vi "Autonomous Independent.vi"() -> ()   [LabVIEW 2020]
doc: "This VI is called when autonomous begins, and will automatically be terminated when autonomous ends. You can carry out timed or sensor driven robot movement independently without needing to return to the caller."
uses:
  <vilib>/Rock Robotics/WPI/Solenoid/WPI_SolenoidValue.ctl
  <vilib>/Rock Robotics/WPI/Utilities/WPI_GetSetVariantRefNum.vi
  <vilib>/Rock Robotics/Network Tables/NT Write Numeric Array.vi
  <vilib>/Rock Robotics/WPI/Solenoid/WPI_SolenoidSetEnum.vi
  Robot Global Data.vi
  <vilib>/Rock Robotics/WPI/RobotDrive/WPI_RobotDriveArcadeDrive_Standard(NoSaturation).vi
  <vilib>/Rock Robotics/Network Tables/NT Read String.vi
panel:
  out "Current Movement, for debugging":T1 {"Y Joystick Value" scale=1.0..-1.0; "X Joystick Value" scale=-1.0..1.0}
  in  "Array of robot movements":T2(array[cluster])=[{"X Joystick Value"=0.39393939393939403, "Y Joystick Value"=0.0, "Delay (sec)"=1.0, "Movement Name"="turn"}, {"X Joystick Value"=-0.3737373737373737, "Y Joystick Value"=0.0, "Delay (sec)"=1.0, "Movement Name"="turn back"}] {"Y Joystick Value" scale=1.0..-1.0; "X Joystick Value" scale=-1.0..1.0}
  # "Be sure to right-click and choose Data Operations>>Make Current Value default if you want to save the array values with the VI"
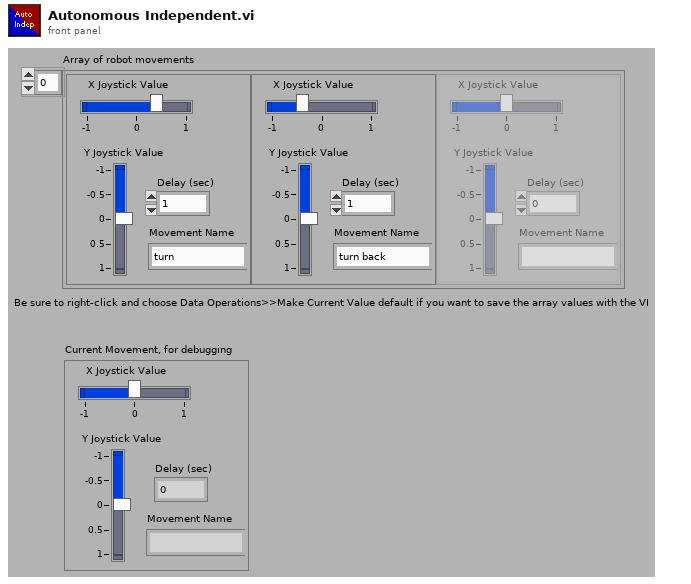
[diagram p1: front panel]
types:
  T1 = cluster{"X Joystick Value":dbl, "Y Joystick Value":dbl, "Delay (sec)":dbl, "Movement Name":string}
  T2 = cluster{"X Joystick Value":dbl, "Y Joystick Value":dbl, "Delay (sec)":dbl, "Movement Name":string}[]
  T3 = typedef "WPI_JoystickDevRef.ctl" = cluster{"Device":T4}
  T4 = typedef "WPI_JoystickDeviceEnum.ctl" = enum16{"USB 0", "USB 1", "USB 2", "USB 3", "USB 4", "USB 5"}
  T5 = typedef "WPI_SolenoidValue.ctl" = enum16{"Off", "On", "Forward", "Reverse"}
  T6 = typedef "WPI_MotorControlDeviceRef.ctl" = cluster{"DeviceStatus":errorcluster, "Type":T7, "PWM":cluster{"PWM Channel":T8, "DeadBand":T9}, "CAN":cluster{"Device Number":u8, "SetOutput VI Ref":variant, "GetOutput VI Ref":variant, "Enable VI Ref":variant, "Disable VI Ref":variant, "Data":variant}, "Invert":bool, "DIO PWM":cluster{"PWM \"Enable\" Channel":T8, "DIOChannel":T10, "PWM Rate":dbl}}
  T7 = typedef "WPI_MotorControlType.ctl" = enum16{"PWM", "CAN", "DIO PWM"}
  T8 = typedef "FPGA_DIOPWMChannel.ctl" = enum8{"PWM 0", "PWM 1", "PWM 2", "PWM 3", "PWM 4", "PWM 5", "PWM 6", "PWM 7", "PWM 8", "PWM 9", "PWM MXP 0", "PWM MXP 1", "PWM MXP 2", "PWM MXP 3", "PWM MXP 4", "PWM MXP 5", "PWM MXP 6", "PWM MXP 7", "PWM MXP 8", "PWM MXP 9", "Invalid"}
  T9 = typedef "WPI_PWMDeadband.ctl" = cluster{"Name":string, "maxPositivePwm":i32, "minPositivePwm":i32, "centerPwm":i32, "maxNegativePwm":i32, "minNegativePwm":i32, "angularRange":u16}
  T10 = typedef "FPGA_DIOChannel.ctl" = enum8{"DIO 0", "DIO 1", "DIO 2", "DIO 3", "DIO 4", "DIO 5", "DIO 6", "DIO 7", "DIO 8", "DIO 9", "DIO MXP 0", "DIO MXP 1", "DIO MXP 2", "DIO MXP 3", "DIO MXP 4", "DIO MXP 5", "DIO MXP 6", "DIO MXP 7", "DIO MXP 8", "DIO MXP 9", "DIO MXP 10", "DIO MXP 11", "DIO MXP 12", "DIO MXP 13", "DIO MXP 14", "DIO MXP 15", "SPI Port CS1", "SPI Port CS2", "SPI Port CS3", "SPI Port MISO", "SPI Port MOSI", "Invalid"}
  T11 = typedef "WPI_SolenoidDevRef.ctl" = cluster{"DevStatus":errorcluster, "Pneumatics Control Module":u8, "Forward Solenoid Channel":T12, "Reverse Solenoid Channel":T12}
  T12 = typedef "WPI_SolenoidChannel.ctl" = enum8{"Solenoid 0", "Solenoid 1", "Solenoid 2", "Solenoid 3", "Solenoid 4", "Solenoid 5", "Solenoid 6", "Solenoid 7", "Solenoid 8", "Solenoid 9", "Solenoid 10", "Solenoid 11", "Solenoid 12", "Solenoid 13", "Solenoid 14", "Solenoid 15", "Invalid"}
  T13 = typedef "WPI_RobotDriveDevRef.ctl" = cluster{"DevStatus":errorcluster, "Motors[]":T6[], "Square Inputs":bool, "Max Output":dbl}
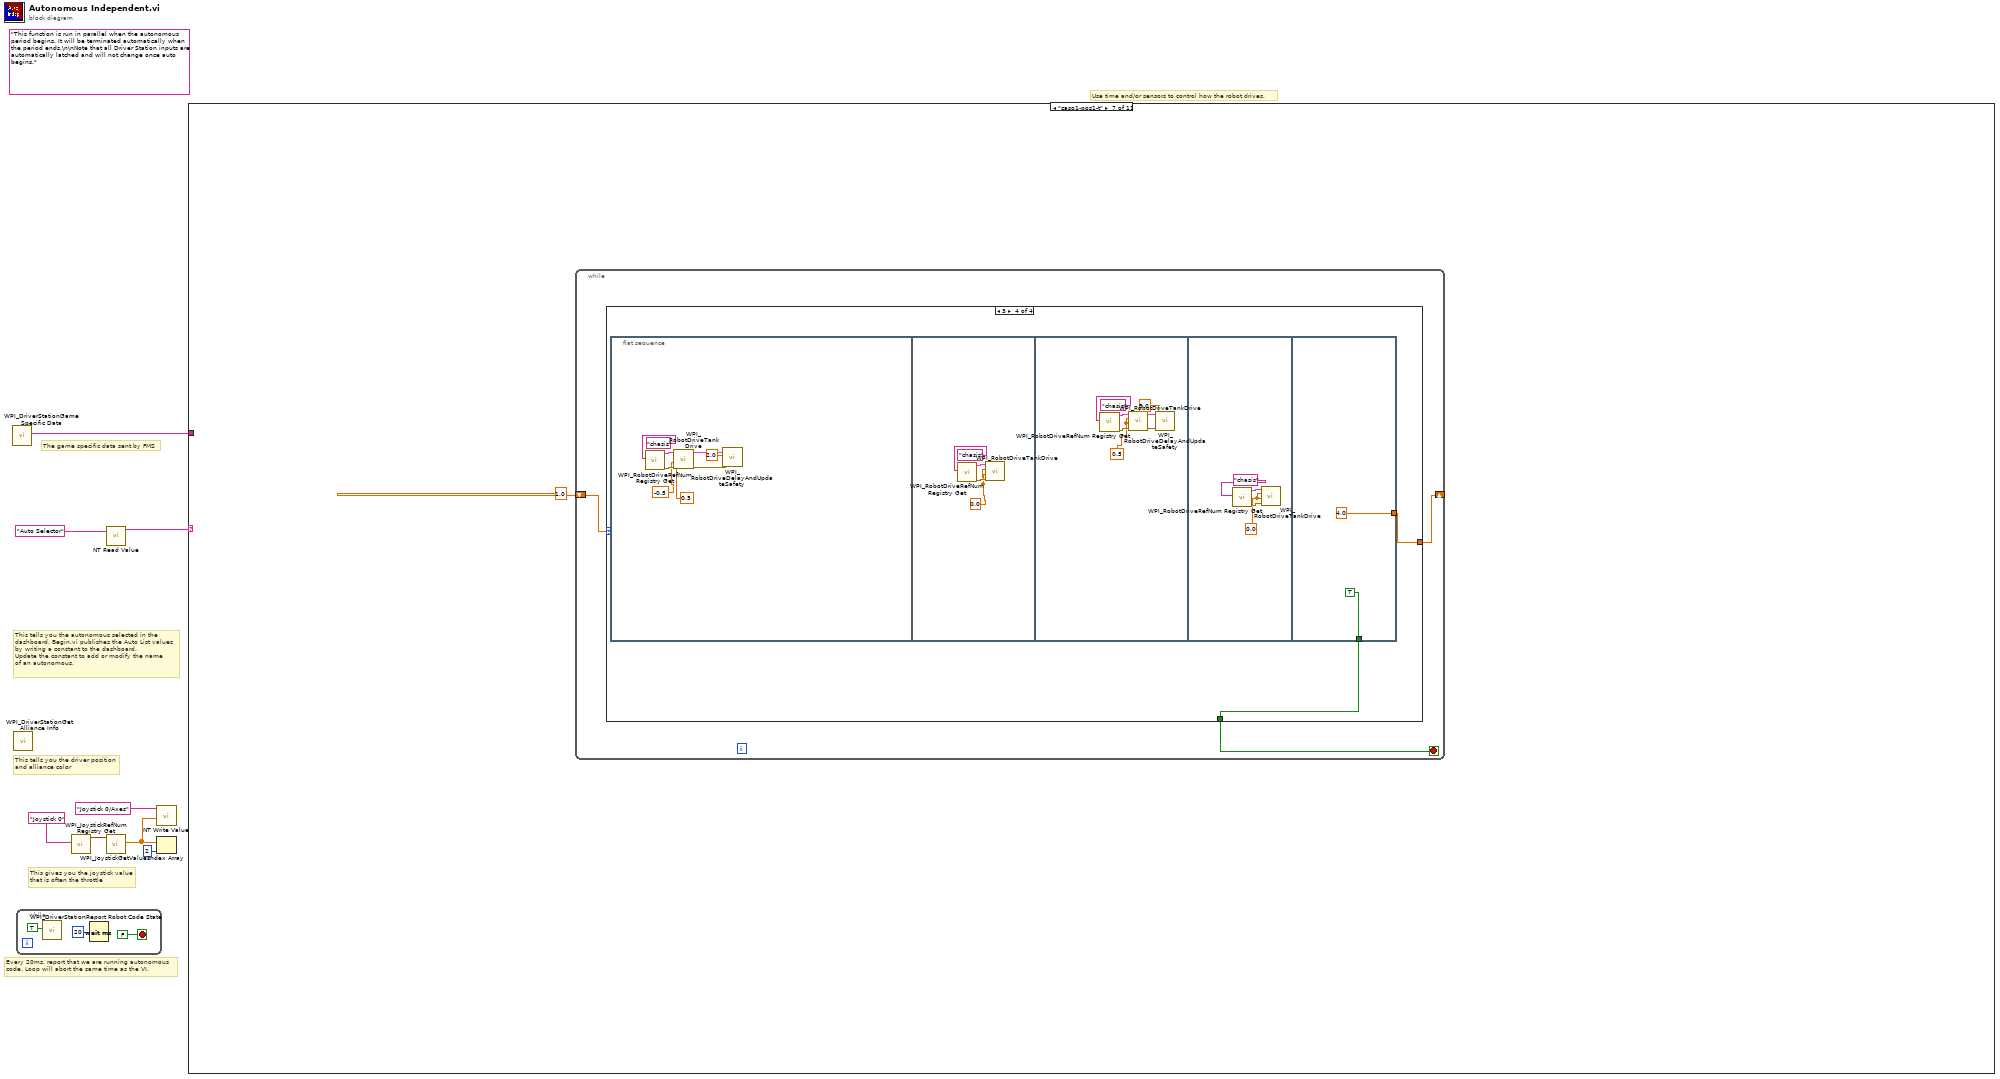
[diagram p0: block diagram]
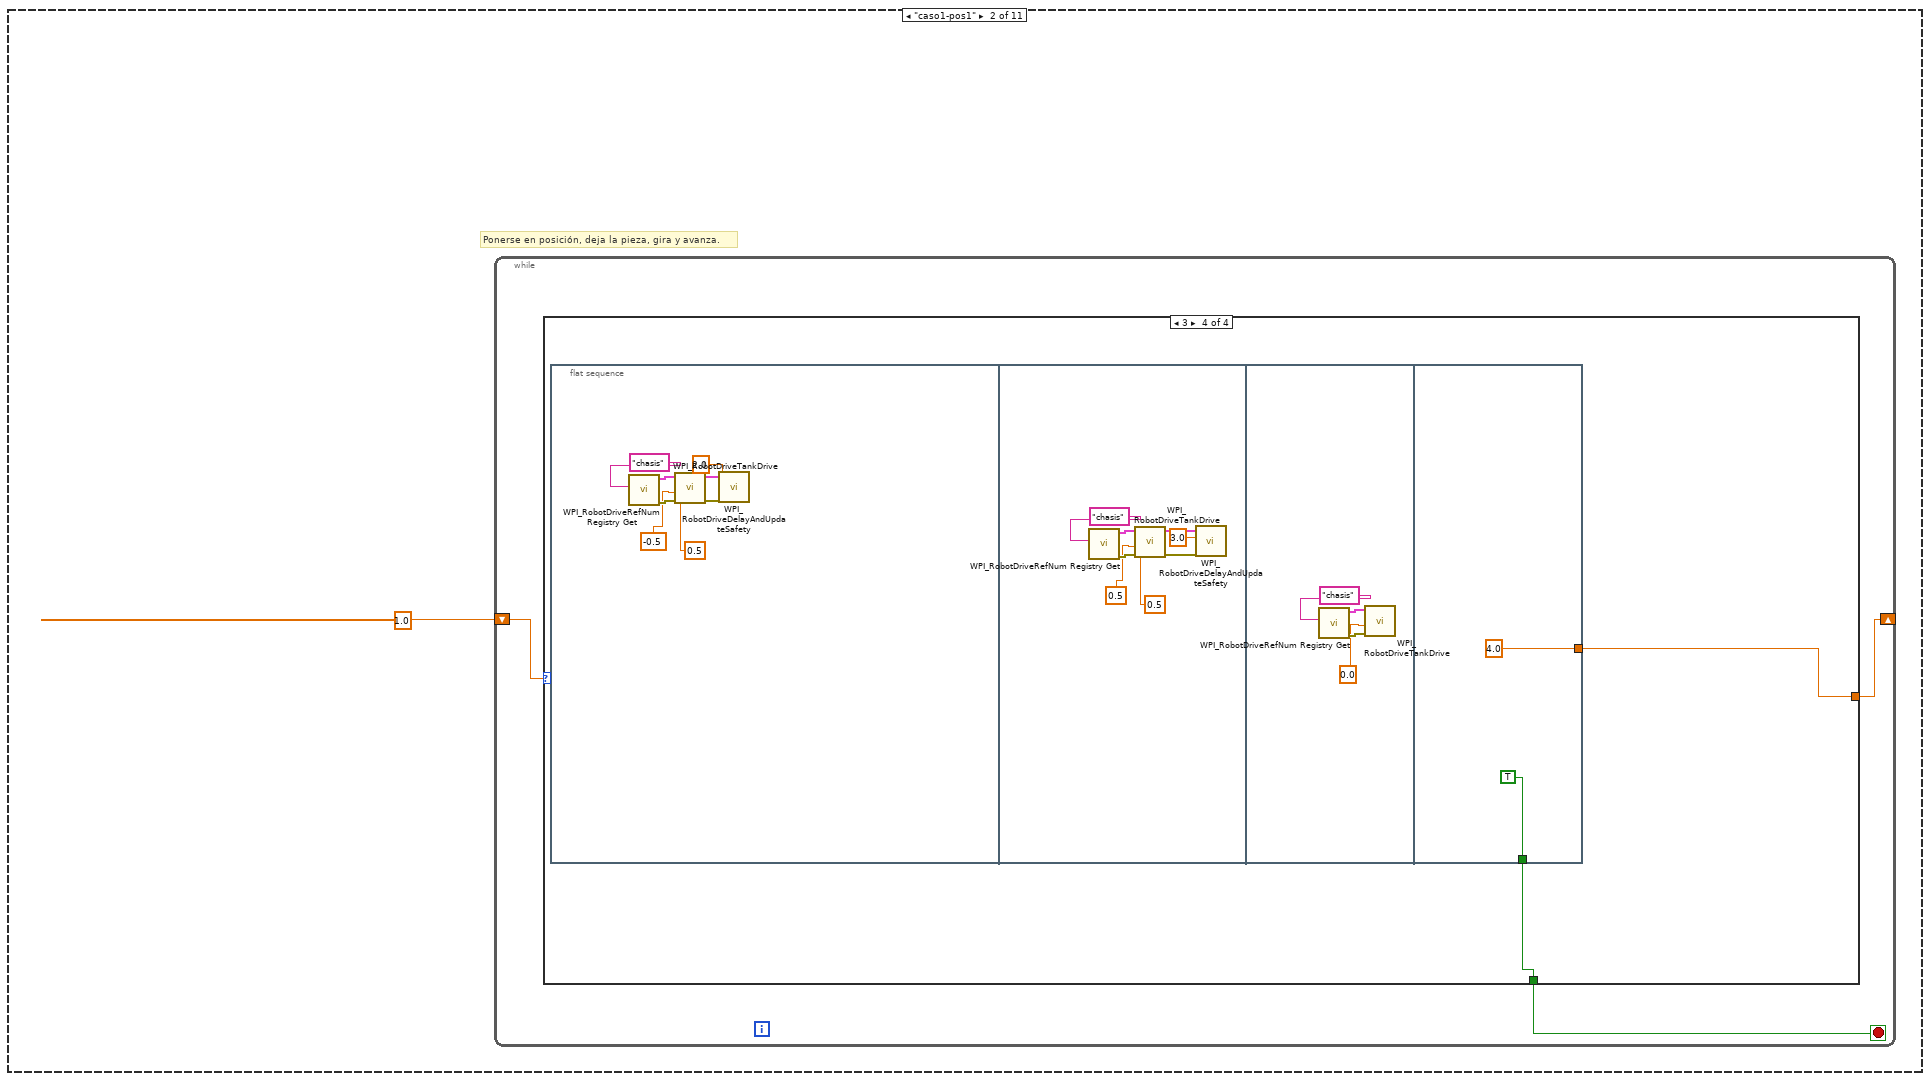
[diagram p3: hidden frame]
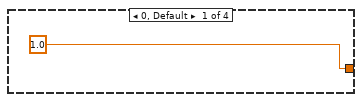
[diagram p4: hidden frame]
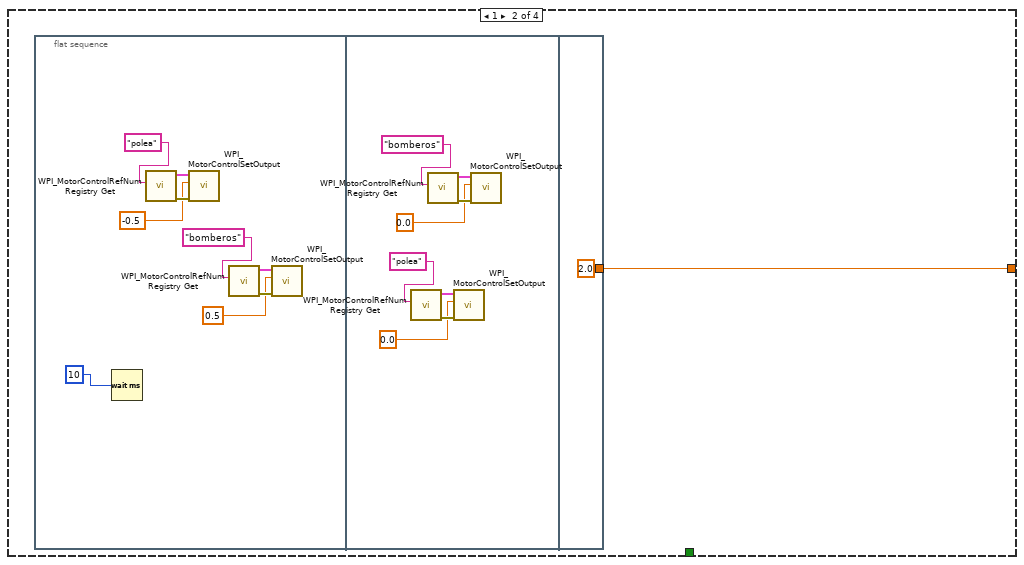
[diagram p5: hidden frame]
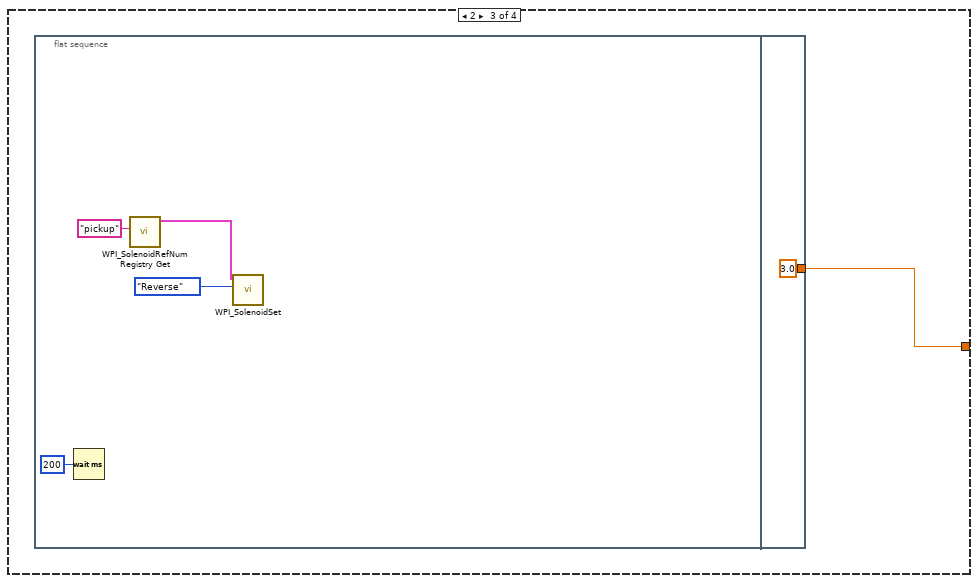
[diagram p6: hidden frame]
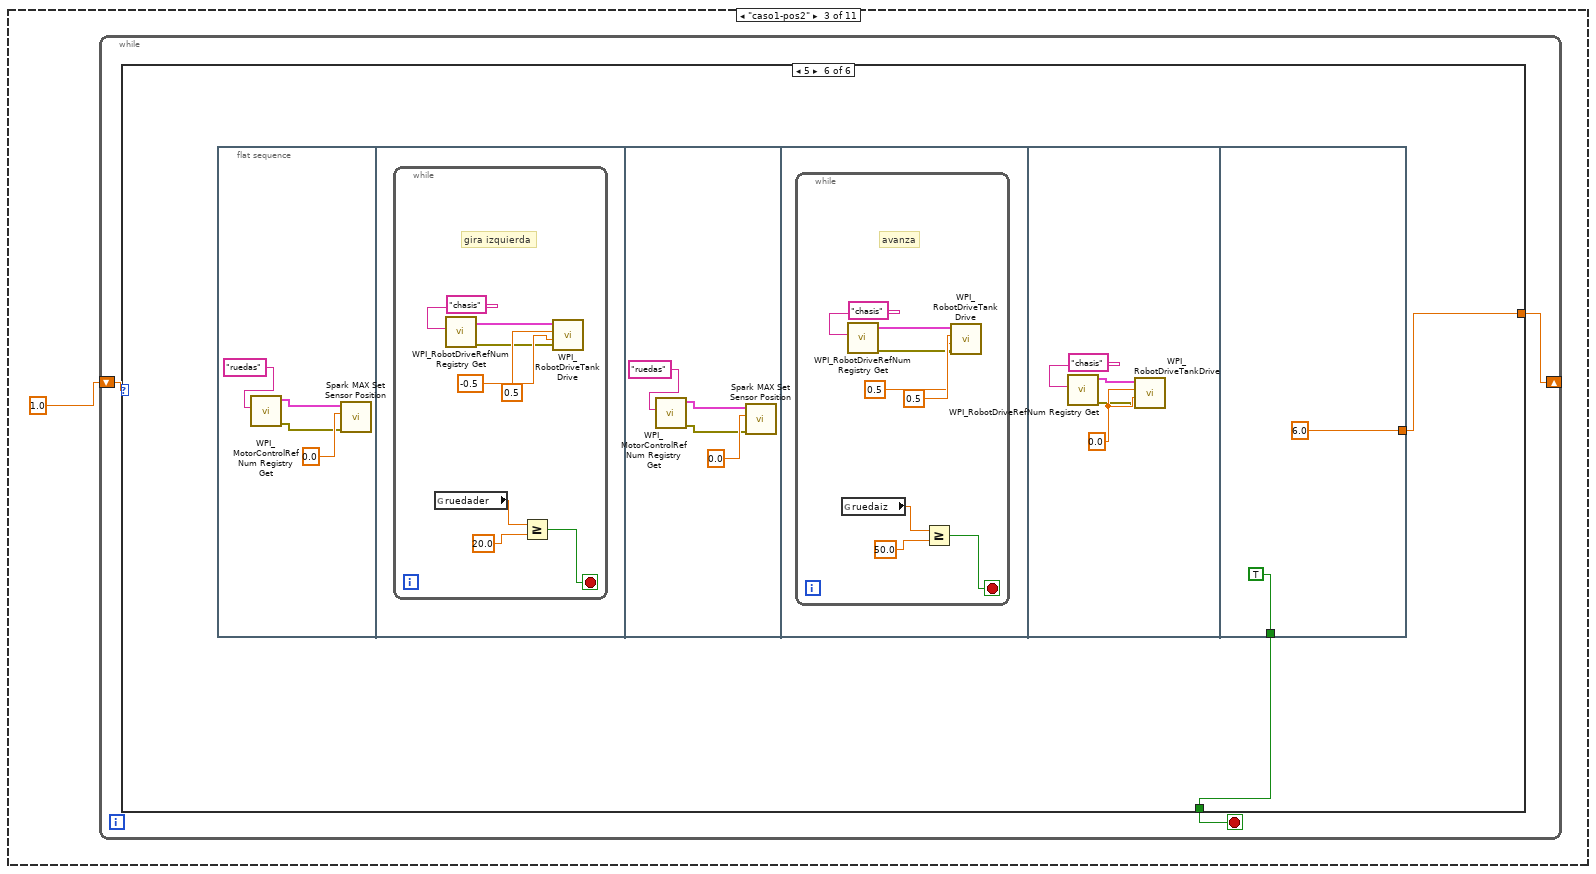
[diagram p7: hidden frame]
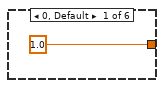
[diagram p8: hidden frame]
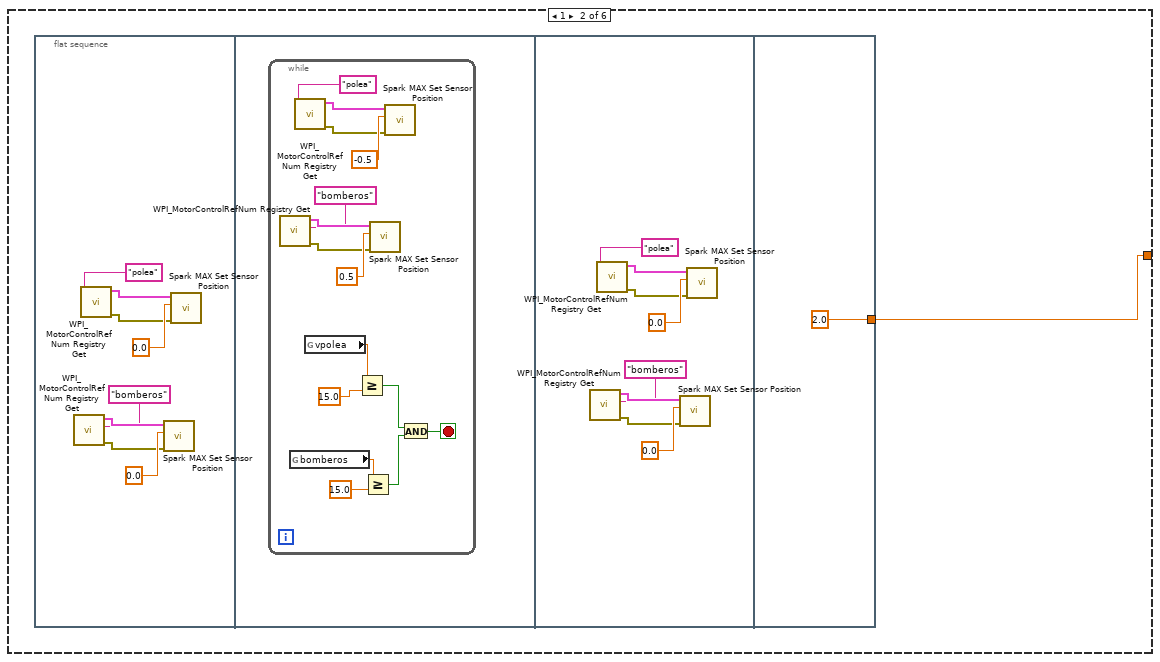
[diagram p9: hidden frame]
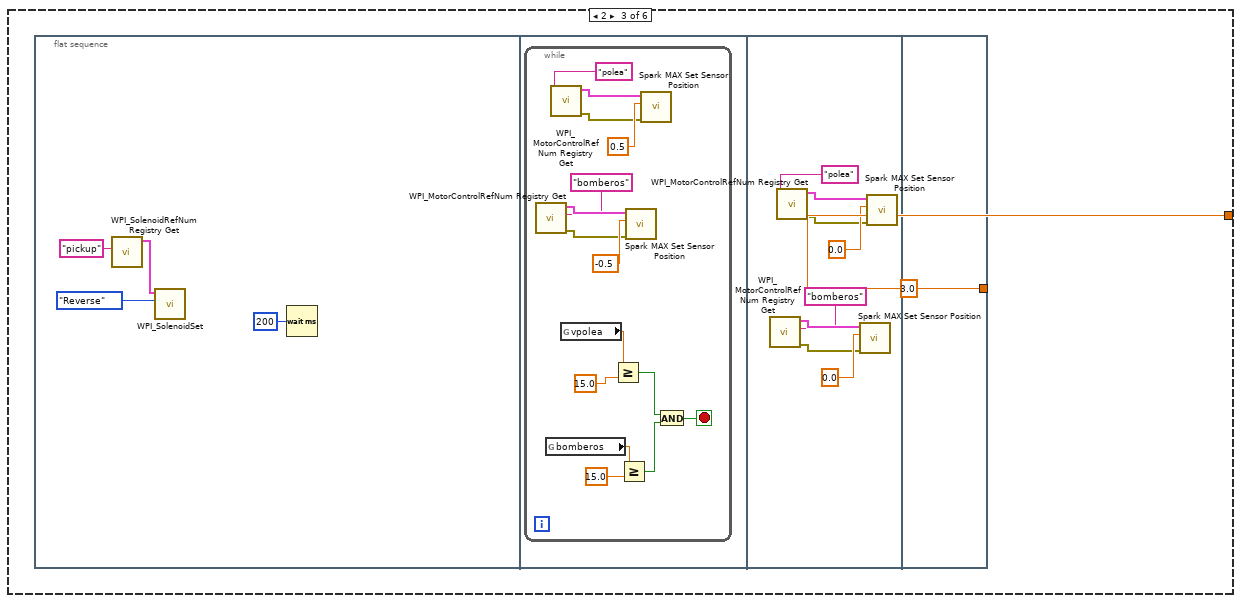
[diagram p10: hidden frame]
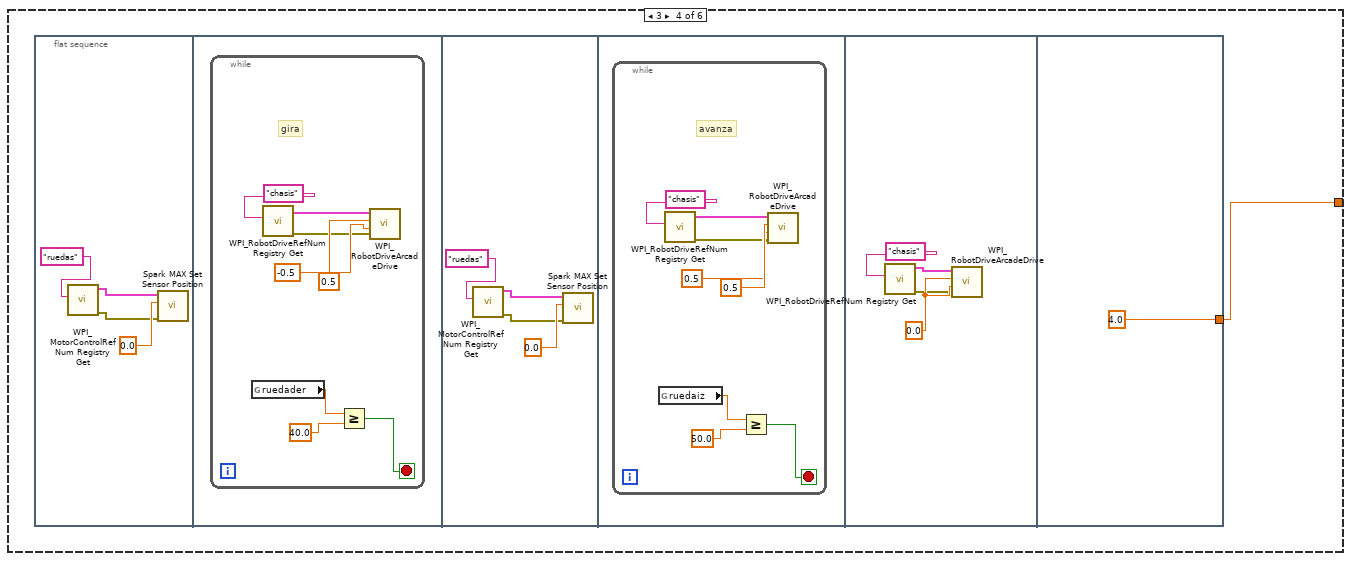
[diagram p11: hidden frame]
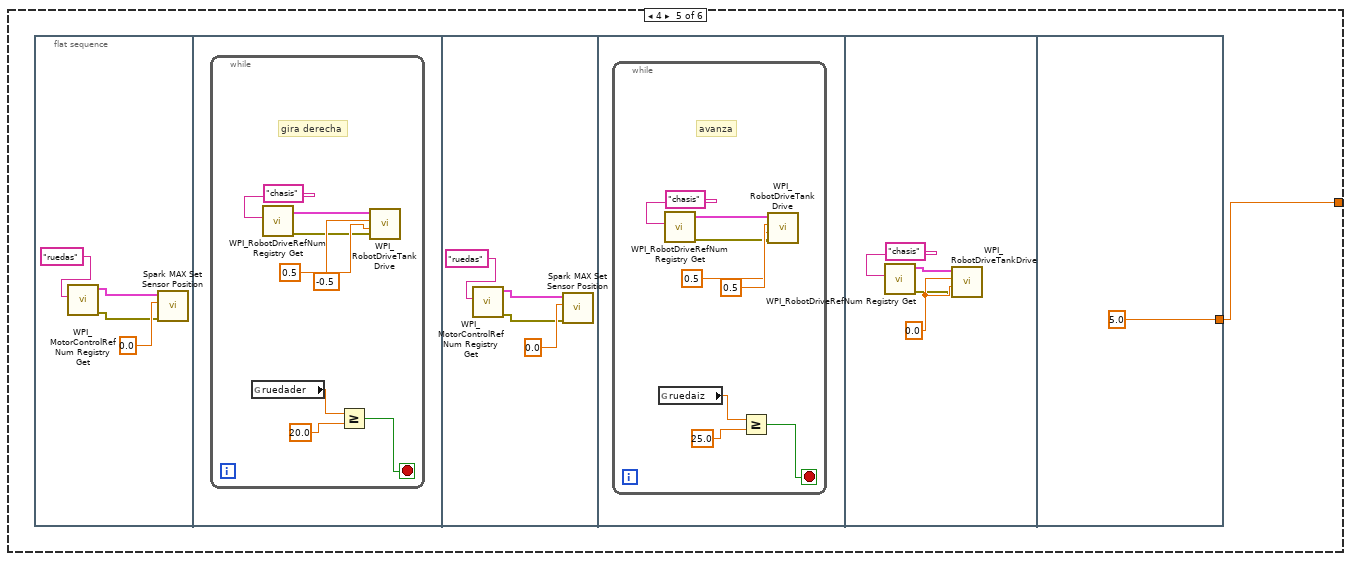
[diagram p12: hidden frame]
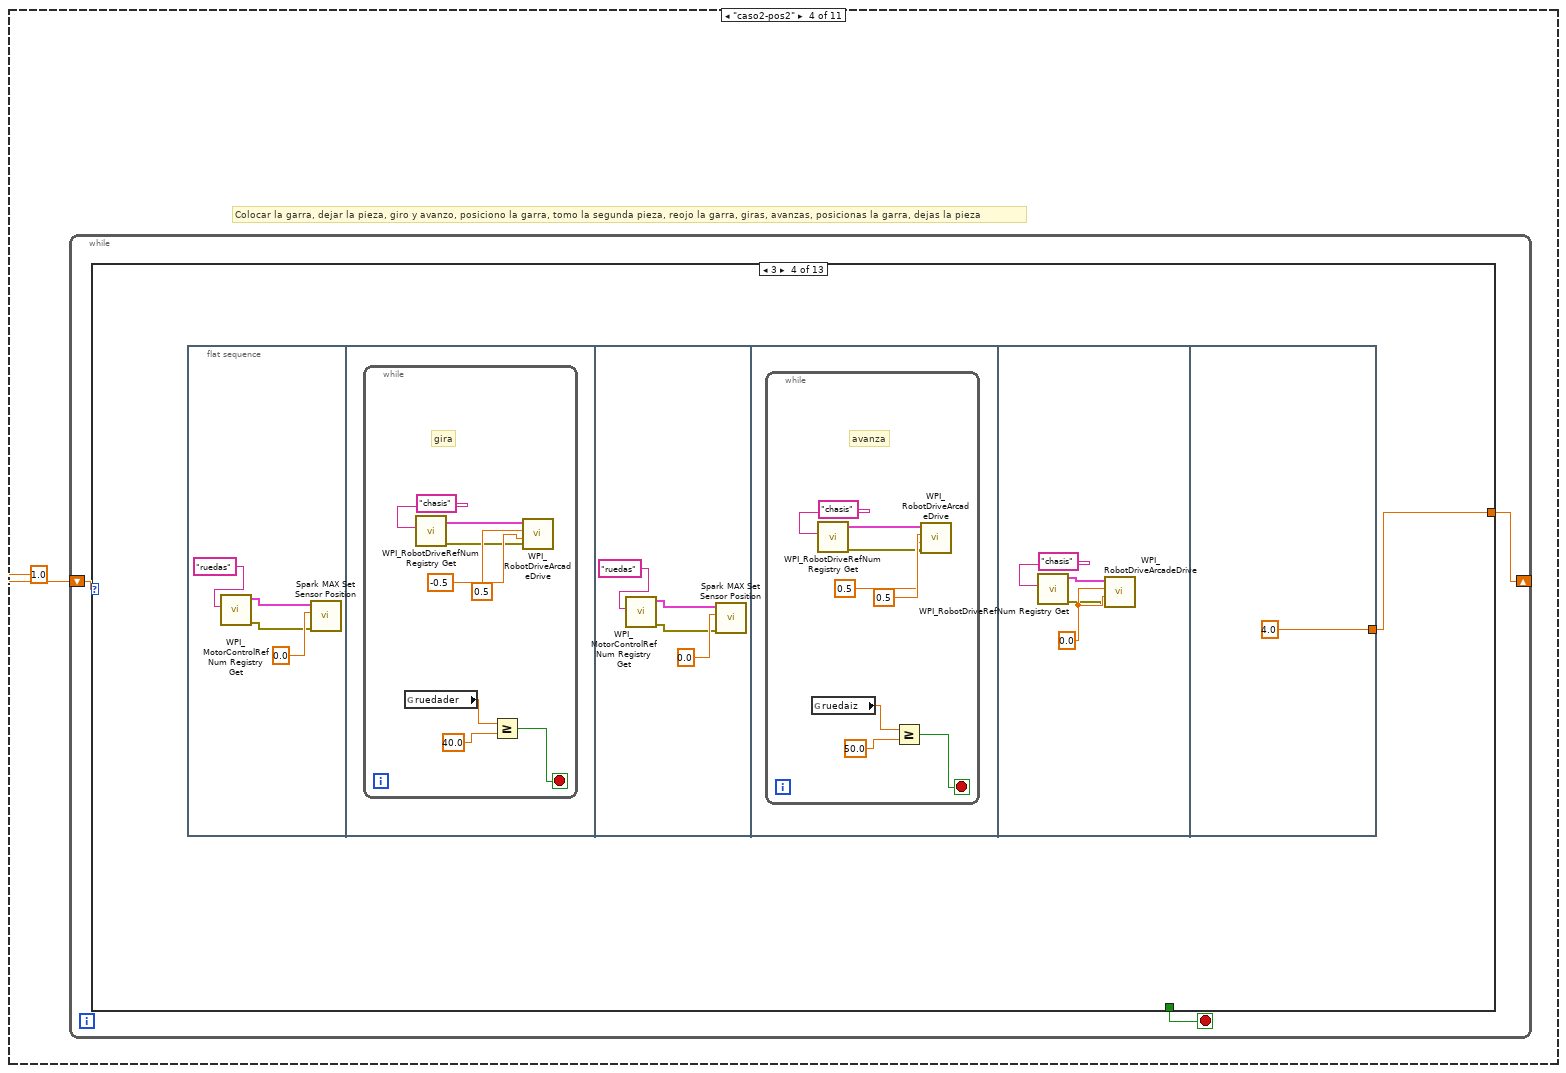
[diagram p13: hidden frame]
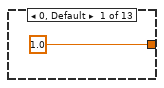
[diagram p14: hidden frame]
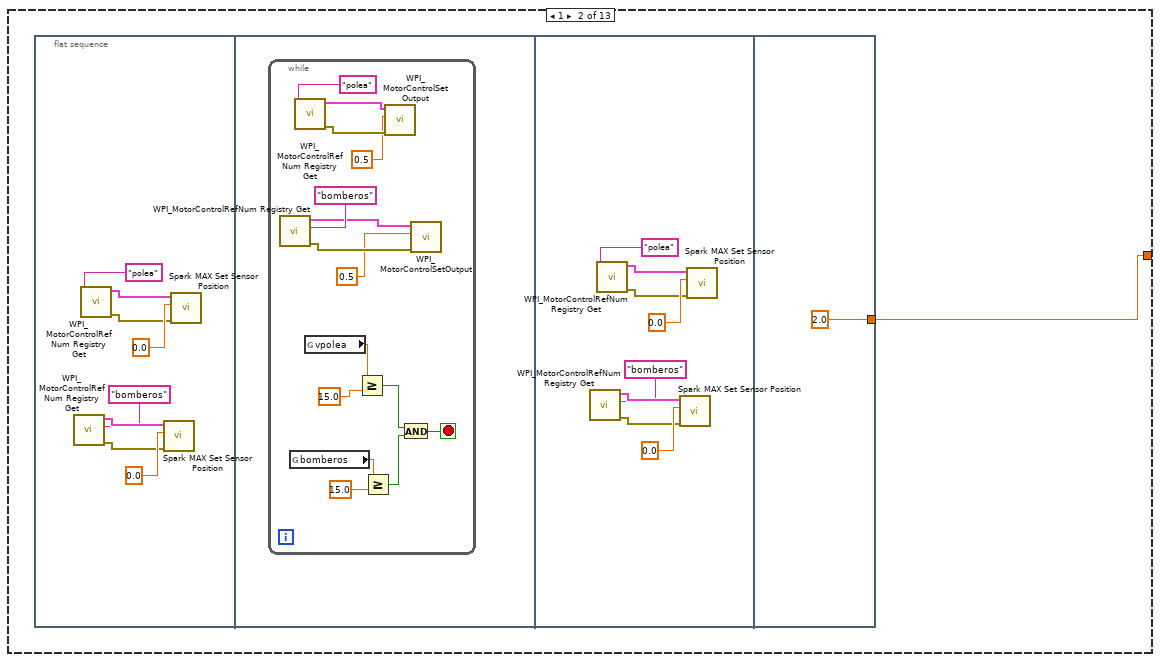
[diagram p15: hidden frame]
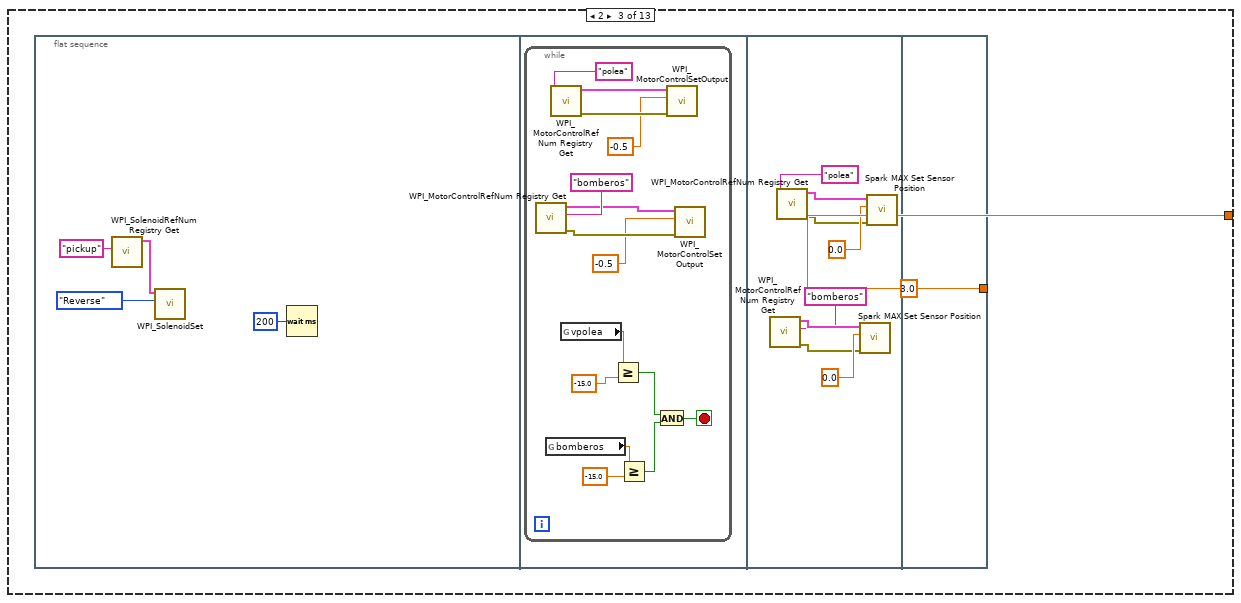
[diagram p16: hidden frame]
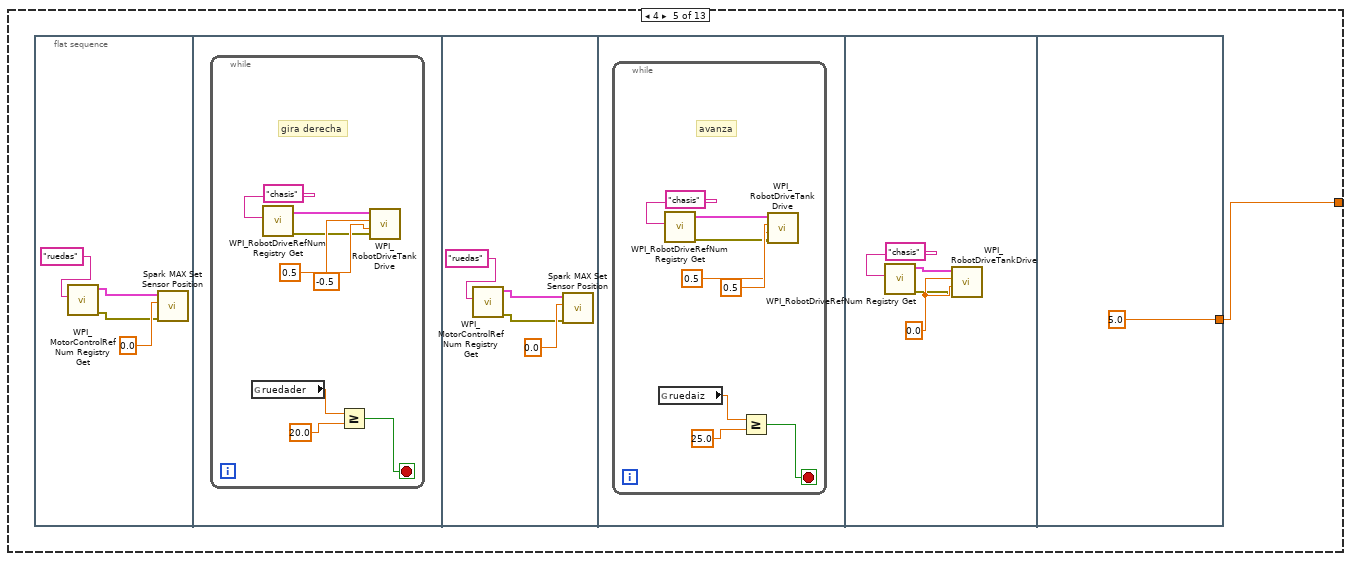
[diagram p17: hidden frame]
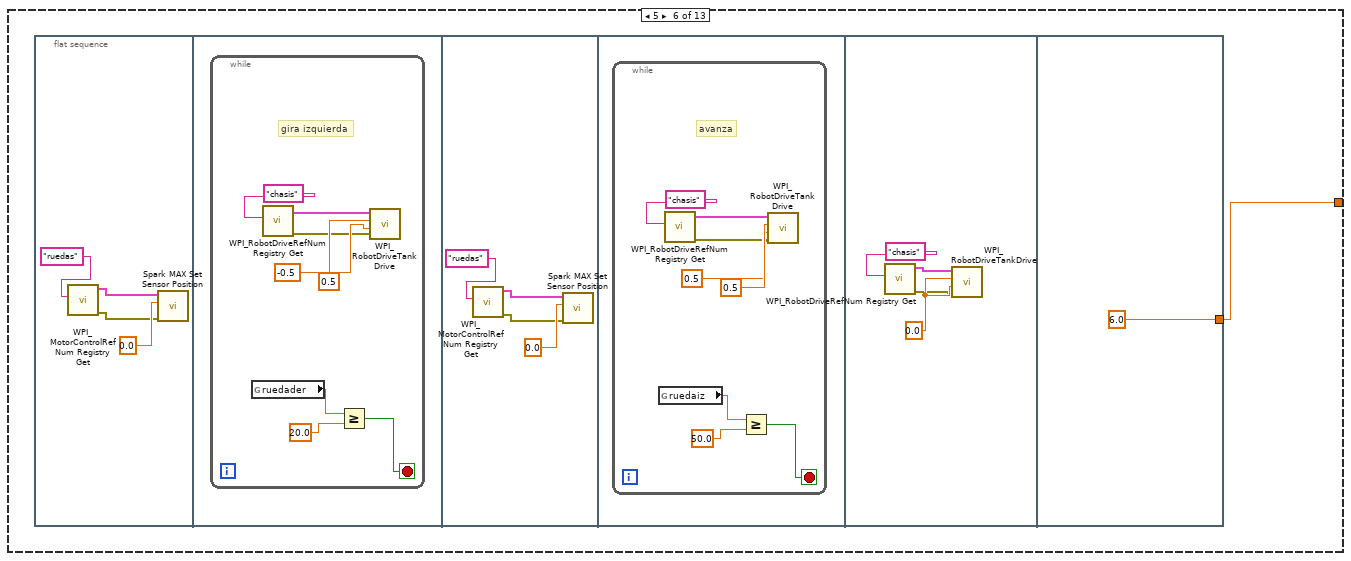
[diagram p18: hidden frame]
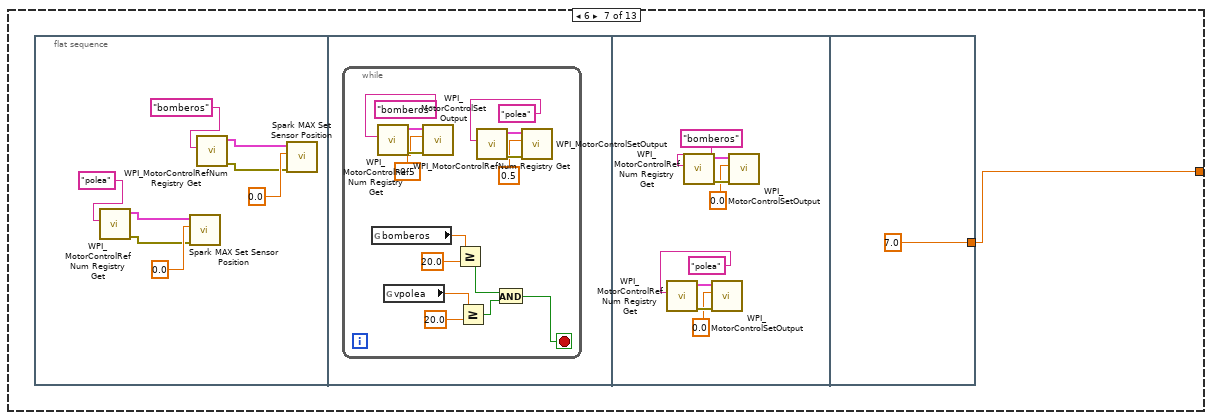
[diagram p19: hidden frame]
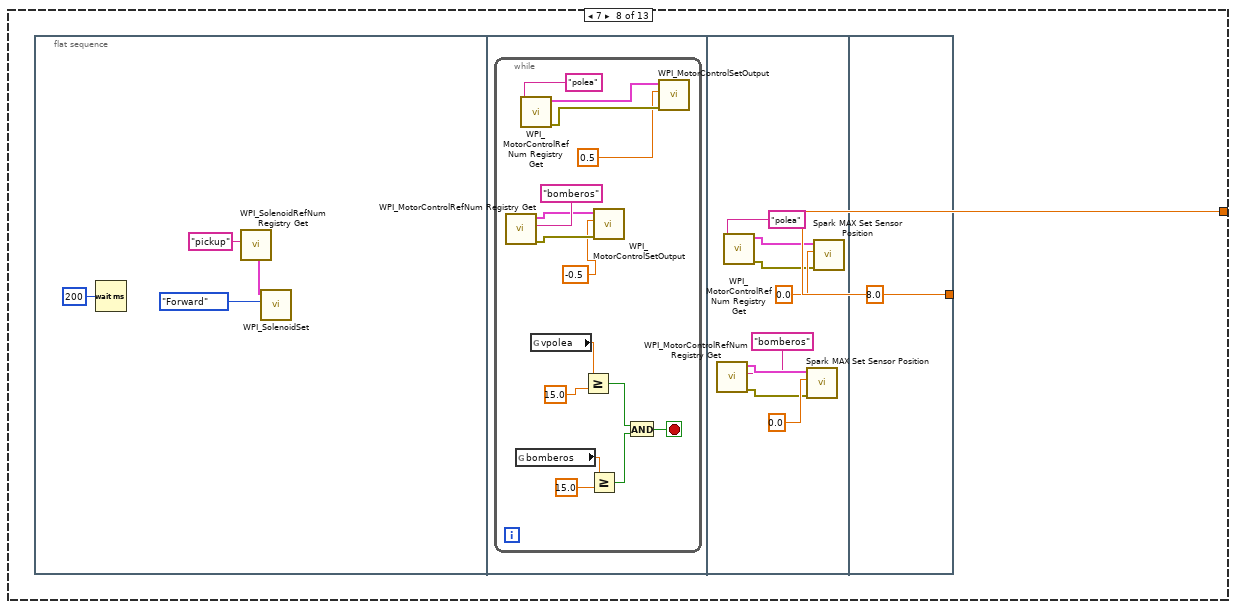
[diagram p20: hidden frame]
diagram:
  (unwired) "This function is run in parallel when the autonomous period begins. It will be terminated automatically when the period ends.\n\nNote that all Driver Station inputs are automatically latched and will not change once auto begins."
  # "The game specific data sent by FMS"
  # "This tells you the autonomous selected in the \ndashboard. Begin.vi publishes the Auto List values\nby writing a constant to the dashboard.\nUpdate the constant to add or modify the name\nof an autonomous."
  # "Every 20ms, report that we are running autonomous\ncode. Loop will abort the same time as the VI."
  # "This gives you the joystick value\nthat is often the throttle"
  # "Use time and/or sensors to control how the robot drives."
  # "This tells you the driver position\nand alliance color"
  n1 = call <vilib>:"WPI_DriverStationGame Specific Data.vi"() -> ("Game Specific Data"=w1:string)  [unwired: 11 in]
  n2 = call <vilib>:"WPI_DriverStationGet Alliance Info.vi"() -> ()  [unwired: 12 out]
  n3 = while {
    stop <- FALSE stop-if-true
    n4 = call <vilib>:"WPI_DriverStationReport Robot Code State.vi"("Autonomous"=TRUE) -> ()  [unwired: 10 in, 1 out]
    n5 = Wait (ms)(milliseconds to wait=u32 20) -> ()  [unwired: 1 out]
  }
  n6 = call <vilib>:"WPI_JoystickRefNum Registry Get.vi"("refnum name"="Joystick 0") -> ("JoystickDevRef"=w7:T3)  [unwired: 1 in, 9 out]
  n7 = call <vilib>:"WPI_JoystickGetValues.vi"("JoystickDevRef"=w7) -> ("Axes"=w3:dbl[])  [unwired: 6 in, 4 out]
  n8 = call-poly <vilib>:"NT Read Value.vi"("Name"="Auto Selector") -> ("String"=w4:string)  [unwired: 9 in, 1 out]
  n9 = call-poly <vilib>:"NT Write Value.vi"("Numeric Array"=w3, "Name"="Joystick 0/Axes") -> ()  [unwired: 9 in, 1 out]
  n10 = Index Array(array=w3, index=2) -> ()  [unwired: 1 out]
  n11 = case shown="\"caso1-pos1-t\"" w4 {
    tunnel: w1 -> [_ _ _ _ _ _ _ _ _ _ _]
    frame Default {
      # "You can put your main auto here, or you can right-click on the case and make any\nother frame be the default case."
      # "This is the frame that will execute if no selection is made, or if it is not recognized"
    }
    frame "caso1-pos1" {
      # "Ponerse en posición, deja la pieza, gira y avanza."
      n12 = while {
        shift-right: [w15] -> _
        shift-left: 1.0 -> [w13]
        stop <- w14 stop-if-true
        n13 = case shown="3" w13 {
          tunnel: [1.0 w17 w36 w43] -> w15
          tunnel: [_ _ _ w42] -> w14
          frame 0, Default {
          }
          frame 1 {
            n14 = flat-sequence {
              tunnel: [2.0] -> w17
              frame #0 {
                n15 = Wait (ms)(milliseconds to wait=u32 10 ("millisecond timer value")) -> ()  [unwired: 1 out]
                n16 = call <vilib>:"WPI_MotorControlRefNum Registry Get.vi"("refnum name"="polea") -> ("error out"=w26:errorcluster, "MotorControlDevRef"=w25:T6)  [unwired: 9 in]
                n17 = call <vilib>:"WPI_MotorControlSetOutput.vi"("error in (no error)"=w26, "Output"=-0.5, "MotorControlDevRef"=w25) -> ()  [unwired: 6 in, 3 out]
                n18 = call <vilib>:"WPI_MotorControlRefNum Registry Get.vi"("refnum name"="bomberos") -> ("error out"=w22:errorcluster, "MotorControlDevRef"=w21:T6)  [unwired: 9 in]
                n19 = call <vilib>:"WPI_MotorControlSetOutput.vi"("error in (no error)"=w22, "Output"=0.5, "MotorControlDevRef"=w21) -> ()  [unwired: 6 in, 3 out]
              }
              frame #1 {
                n20 = call <vilib>:"WPI_MotorControlRefNum Registry Get.vi"("refnum name"="polea") -> ("error out"=w33:errorcluster, "MotorControlDevRef"=w34:T6)  [unwired: 9 in]
                n21 = call <vilib>:"WPI_MotorControlRefNum Registry Get.vi"("refnum name"="bomberos") -> ("error out"=w29:errorcluster, "MotorControlDevRef"=w30:T6)  [unwired: 9 in]
                n22 = call <vilib>:"WPI_MotorControlSetOutput.vi"("error in (no error)"=w33, "Output"=0.0, "MotorControlDevRef"=w34) -> ()  [unwired: 6 in, 3 out]
                n23 = call <vilib>:"WPI_MotorControlSetOutput.vi"("error in (no error)"=w29, "Output"=0.0, "MotorControlDevRef"=w30) -> ()  [unwired: 6 in, 3 out]
              }
              frame #2 {
              }
            }
          }
          frame 2 {
            n24 = flat-sequence {
              tunnel: [3.0] -> w36
              frame #0 {
                n25 = Wait (ms)(milliseconds to wait=u32 200) -> ()  [unwired: 1 out]
                n26 = call <vilib>:"WPI_SolenoidRefNum Registry Get.vi"("refnum name"="pickup") -> ("SolenoidDevRef"=w40:T11)  [unwired: 9 in, 1 out]
                n27 = call-poly <vilib>:"WPI_SolenoidSet.vi"("Value"=WPI_SolenoidValue."Reverse", "SolenoidDevRef"=w40) -> ()  [unwired: 8 in, 2 out]
              }
              frame #1 {
              }
            }
          }
          frame 3 {
            n28 = flat-sequence {
              tunnel: [4.0] -> w43
              tunnel: [TRUE] -> w42
              frame #0 {
                n29 = call <vilib>:"WPI_RobotDriveRefNum Registry Get.vi"("refnum name"="chasis") -> ("error out"=w51:errorcluster, "RobotDriveDevRef"=w50:T13)  [unwired: 9 in]
                n30 = call <vilib>:"WPI_RobotDriveTankDrive.vi"("error in (no error)"=w51, "Right axis value"=-0.5 ("Motor Output"), "Left axis value"=0.5 ("Motor Output"), "RobotDriveDevRef"=w50) -> ("error out"=w46:errorcluster, "RobotDriveDevRef"=w45:T13)  [unwired: 5 in, 1 out]
                n31 = call <vilib>:"WPI_RobotDriveDelayAndUpdateSafety.vi"("error in (no error)"=w46, "Delay (s)"=2.0, "RobotDriveDevRef"=w45) -> ()  [unwired: 7 in, 2 out]
              }
              frame #1 {
                n32 = call <vilib>:"WPI_RobotDriveRefNum Registry Get.vi"("refnum name"="chasis") -> ("error out"=w59:errorcluster, "RobotDriveDevRef"=w58:T13)  [unwired: 9 in]
                n33 = call <vilib>:"WPI_RobotDriveTankDrive.vi"("error in (no error)"=w59, "Right axis value"=0.5 ("Motor Output"), "Left axis value"=0.5 ("Motor Output"), "RobotDriveDevRef"=w58) -> ("error out"=w53:errorcluster, "RobotDriveDevRef"=w54:T13)  [unwired: 5 in, 1 out]
                n34 = call <vilib>:"WPI_RobotDriveDelayAndUpdateSafety.vi"("error in (no error)"=w53, "Delay (s)"=3.0, "RobotDriveDevRef"=w54) -> ()  [unwired: 7 in, 2 out]
              }
              frame #2 {
                n35 = call <vilib>:"WPI_RobotDriveRefNum Registry Get.vi"("refnum name"="chasis") -> ("error out"=w63:errorcluster, "RobotDriveDevRef"=w62:T13)  [unwired: 9 in]
                n36 = call <vilib>:"WPI_RobotDriveTankDrive.vi"("error in (no error)"=w63, "Right axis value"=0.0 ("Motor Output"), "RobotDriveDevRef"=w62) -> ()  [unwired: 6 in, 3 out]
              }
              frame #3 {
              }
            }
          }
        }
      }
    }
    frame "caso1-pos2" {
      n37 = while {
        shift-right: [w68] -> _
        shift-left: 1.0 -> [w69]
        stop <- w67 stop-if-true
        n38 = case shown="5" w69 {
          tunnel: [1.0 w71 w104 w133 w163 w194] -> w68
          tunnel: [_ _ _ _ _ w193] -> w67
          frame 0, Default {
          }
          frame 1 {
            n39 = flat-sequence {
              tunnel: [2.0] -> w71
              frame #0 {
                n40 = call <vilib>:"WPI_MotorControlRefNum Registry Get.vi"("refnum name"="bomberos") -> ("error out"=w74:errorcluster, "MotorControlDevRef"=w75:T6)  [unwired: 9 in]
                n41 = call <vilib>:"WPI_MotorControlRefNum Registry Get.vi"("refnum name"="polea") -> ("error out"=w77:errorcluster, "MotorControlDevRef"=w78:T6)  [unwired: 9 in]
                n42 = call <vilib>:"Spark MAX Set Sensor Position.vi"("error in"=w74, "Position"=0.0, "MotorControlDeviceRef"=w75) -> ()  [unwired: 7 in, 2 out]
                n43 = call <vilib>:"Spark MAX Set Sensor Position.vi"("error in"=w77, "Position"=0.0, "MotorControlDeviceRef"=w78) -> ()  [unwired: 7 in, 2 out]
              }
              frame #1 {
                n44 = while {
                  stop <- w92 stop-if-true
                  n45 = call <vilib>:"WPI_MotorControlRefNum Registry Get.vi"("refnum name"="bomberos") -> ("error out"=w84:errorcluster, "MotorControlDevRef"=w85:T6)  [unwired: 9 in]
                  n46 = global read "Robot Global Data.vi" "bomberos"() -> (w91:dbl)
                  n47 = call <vilib>:"WPI_MotorControlRefNum Registry Get.vi"("refnum name"="polea") -> ("error out"=w87:errorcluster, "MotorControlDevRef"=w88:T6)  [unwired: 9 in]
                  n48 = global read "Robot Global Data.vi" "vpolea"() -> (w94:dbl)
                  n49 = Greater Or Equal?(x=w94, y=15.0) -> (x >= y?=w81:bool)
                  n50 = Greater Or Equal?(x=w91, y=15.0) -> (x >= y?=w80:bool)
                  n51 = call <vilib>:"Spark MAX Set Sensor Position.vi"("error in"=w84, "Position"=0.5, "MotorControlDeviceRef"=w85) -> ()  [unwired: 7 in, 2 out]
                  n52 = call <vilib>:"Spark MAX Set Sensor Position.vi"("error in"=w87, "Position"=-0.5, "MotorControlDeviceRef"=w88) -> ()  [unwired: 7 in, 2 out]
                  n53 = And(x=w81, y=w80) -> (x .and. y?=w92:bool)
                }
              }
              frame #2 {
                n54 = call <vilib>:"WPI_MotorControlRefNum Registry Get.vi"("refnum name"="bomberos") -> ("error out"=w97:errorcluster, "MotorControlDevRef"=w98:T6)  [unwired: 9 in]
                n55 = call <vilib>:"WPI_MotorControlRefNum Registry Get.vi"("refnum name"="polea") -> ("error out"=w100:errorcluster, "MotorControlDevRef"=w101:T6)  [unwired: 9 in]
                n56 = call <vilib>:"Spark MAX Set Sensor Position.vi"("error in"=w97, "Position"=0.0, "MotorControlDeviceRef"=w98) -> ()  [unwired: 7 in, 2 out]
                n57 = call <vilib>:"Spark MAX Set Sensor Position.vi"("error in"=w100, "Position"=0.0, "MotorControlDeviceRef"=w101) -> ()  [unwired: 7 in, 2 out]
              }
              frame #3 {
              }
            }
          }
          frame 2 {
            n58 = flat-sequence {
              tunnel: [3.0] -> w104
              frame #0 {
                n59 = call <vilib>:"WPI_SolenoidRefNum Registry Get.vi"("refnum name"="pickup") -> ("SolenoidDevRef"=w105:T11)  [unwired: 9 in, 1 out]
                n60 = call-poly <vilib>:"WPI_SolenoidSet.vi"("Value"=WPI_SolenoidValue."Reverse", "SolenoidDevRef"=w105) -> ()  [unwired: 8 in, 2 out]
                n61 = Wait (ms)(milliseconds to wait=u32 200) -> ()  [unwired: 1 out]
              }
              frame #1 {
                n62 = while {
                  stop <- w121 stop-if-true
                  n63 = call <vilib>:"WPI_MotorControlRefNum Registry Get.vi"("refnum name"="bomberos") -> ("error out"=w113:errorcluster, "MotorControlDevRef"=w114:T6)  [unwired: 9 in]
                  n64 = global read "Robot Global Data.vi" "bomberos"() -> (w120:dbl)
                  n65 = call <vilib>:"WPI_MotorControlRefNum Registry Get.vi"("refnum name"="polea") -> ("error out"=w116:errorcluster, "MotorControlDevRef"=w117:T6)  [unwired: 9 in]
                  n66 = global read "Robot Global Data.vi" "vpolea"() -> (w123:dbl)
                  n67 = Greater Or Equal?(x=w123, y=15.0) -> (x >= y?=w110:bool)
                  n68 = Greater Or Equal?(x=w120, y=15.0) -> (x >= y?=w109:bool)
                  n69 = call <vilib>:"Spark MAX Set Sensor Position.vi"("error in"=w113, "Position"=-0.5, "MotorControlDeviceRef"=w114) -> ()  [unwired: 7 in, 2 out]
                  n70 = call <vilib>:"Spark MAX Set Sensor Position.vi"("error in"=w116, "Position"=0.5, "MotorControlDeviceRef"=w117) -> ()  [unwired: 7 in, 2 out]
                  n71 = And(x=w110, y=w109) -> (x .and. y?=w121:bool)
                }
              }
              frame #2 {
                n72 = call <vilib>:"WPI_MotorControlRefNum Registry Get.vi"("refnum name"="bomberos") -> ("error out"=w126:errorcluster, "MotorControlDevRef"=w127:T6)  [unwired: 9 in]
                n73 = call <vilib>:"WPI_MotorControlRefNum Registry Get.vi"("refnum name"="polea") -> ("error out"=w129:errorcluster, "MotorControlDevRef"=w130:T6)  [unwired: 9 in]
                n74 = call <vilib>:"Spark MAX Set Sensor Position.vi"("error in"=w126, "Position"=0.0, "MotorControlDeviceRef"=w127) -> ()  [unwired: 7 in, 2 out]
                n75 = call <vilib>:"Spark MAX Set Sensor Position.vi"("error in"=w129, "Position"=0.0, "MotorControlDeviceRef"=w130) -> ()  [unwired: 7 in, 2 out]
              }
              frame #3 {
              }
            }
          }
          frame 3 {
            n76 = flat-sequence {
              tunnel: [4.0] -> w133
              frame #0 {
                n77 = call <vilib>:"WPI_MotorControlRefNum Registry Get.vi"("refnum name"="ruedas") -> ("error out"=w134:errorcluster, "MotorControlDevRef"=w135:T6)  [unwired: 9 in]
                n78 = call <vilib>:"Spark MAX Set Sensor Position.vi"("error in"=w134, "Position"=0.0, "MotorControlDeviceRef"=w135) -> ()  [unwired: 7 in, 2 out]
              }
              frame #1 {
                n79 = while {
                  stop <- w142 stop-if-true
                  # "gira"
                  n80 = global read "Robot Global Data.vi" "ruedader"() -> (w144:dbl)
                  n81 = call <vilib>:"WPI_RobotDriveRefNum Registry Get.vi"("refnum name"="chasis") -> ("error out"=w138:errorcluster, "RobotDriveDevRef"=w139:T13)  [unwired: 9 in]
                  n82 = Greater Or Equal?(x=w144, y=40.0) -> (x >= y?=w142:bool)
                  n83 = call-poly <vilib>:"WPI_RobotDriveArcadeDrive.vi"("error in (no error)"=w138, "Y axis value"=-0.5 ("Motor Output"), "X axis value"=0.5 ("Motor Output"), "RobotDriveDevRef"=w139) -> ()  [unwired: 5 in, 3 out]
                }
              }
              frame #2 {
                n84 = call <vilib>:"WPI_MotorControlRefNum Registry Get.vi"("refnum name"="ruedas") -> ("error out"=w146:errorcluster, "MotorControlDevRef"=w147:T6)  [unwired: 9 in]
                n85 = call <vilib>:"Spark MAX Set Sensor Position.vi"("error in"=w146, "Position"=0.0, "MotorControlDeviceRef"=w147) -> ()  [unwired: 7 in, 2 out]
              }
              frame #3 {
                n86 = while {
                  stop <- w154 stop-if-true
                  # "avanza"
                  n87 = global read "Robot Global Data.vi" "ruedaiz"() -> (w156:dbl)
                  n88 = call <vilib>:"WPI_RobotDriveRefNum Registry Get.vi"("refnum name"="chasis") -> ("error out"=w150:errorcluster, "RobotDriveDevRef"=w151:T13)  [unwired: 9 in]
                  n89 = Greater Or Equal?(x=w156, y=50.0) -> (x >= y?=w154:bool)
                  n90 = call-poly <vilib>:"WPI_RobotDriveArcadeDrive.vi"("error in (no error)"=w150, "Y axis value"=0.5 ("Motor Output"), "X axis value"=0.5 ("Motor Output"), "RobotDriveDevRef"=w151) -> ()  [unwired: 5 in, 3 out]
                }
              }
              frame #4 {
                w160 = 0.0 ("Motor Output")
                n91 = call <vilib>:"WPI_RobotDriveRefNum Registry Get.vi"("refnum name"="chasis") -> ("error out"=w158:errorcluster, "RobotDriveDevRef"=w159:T13)  [unwired: 9 in]
                n92 = call-poly <vilib>:"WPI_RobotDriveArcadeDrive.vi"("error in (no error)"=w158, "Y axis value"=w160, "X axis value"=w160, "RobotDriveDevRef"=w159) -> ()  [unwired: 5 in, 3 out]
              }
              frame #5 {
              }
            }
          }
          frame 4 {
            n93 = flat-sequence {
              tunnel: [5.0] -> w163
              frame #0 {
                n94 = call <vilib>:"WPI_MotorControlRefNum Registry Get.vi"("refnum name"="ruedas") -> ("error out"=w164:errorcluster, "MotorControlDevRef"=w165:T6)  [unwired: 9 in]
                n95 = call <vilib>:"Spark MAX Set Sensor Position.vi"("error in"=w164, "Position"=0.0, "MotorControlDeviceRef"=w165) -> ()  [unwired: 7 in, 2 out]
              }
              frame #1 {
                n96 = while {
                  stop <- w172 stop-if-true
                  # "gira derecha"
                  n97 = global read "Robot Global Data.vi" "ruedader"() -> (w174:dbl)
                  n98 = call <vilib>:"WPI_RobotDriveRefNum Registry Get.vi"("refnum name"="chasis") -> ("error out"=w168:errorcluster, "RobotDriveDevRef"=w169:T13)  [unwired: 9 in]
                  n99 = Greater Or Equal?(x=w174, y=20.0) -> (x >= y?=w172:bool)
                  n100 = call <vilib>:"WPI_RobotDriveTankDrive.vi"("error in (no error)"=w168, "Right axis value"=0.5 ("Motor Output"), "Left axis value"=-0.5 ("Motor Output"), "RobotDriveDevRef"=w169) -> ()  [unwired: 5 in, 3 out]
                }
              }
              frame #2 {
                n101 = call <vilib>:"WPI_MotorControlRefNum Registry Get.vi"("refnum name"="ruedas") -> ("error out"=w176:errorcluster, "MotorControlDevRef"=w177:T6)  [unwired: 9 in]
                n102 = call <vilib>:"Spark MAX Set Sensor Position.vi"("error in"=w176, "Position"=0.0, "MotorControlDeviceRef"=w177) -> ()  [unwired: 7 in, 2 out]
              }
              frame #3 {
                n103 = while {
                  stop <- w184 stop-if-true
                  # "avanza"
                  n104 = global read "Robot Global Data.vi" "ruedaiz"() -> (w186:dbl)
                  n105 = call <vilib>:"WPI_RobotDriveRefNum Registry Get.vi"("refnum name"="chasis") -> ("error out"=w180:errorcluster, "RobotDriveDevRef"=w181:T13)  [unwired: 9 in]
                  n106 = Greater Or Equal?(x=w186, y=25.0) -> (x >= y?=w184:bool)
                  n107 = call <vilib>:"WPI_RobotDriveTankDrive.vi"("error in (no error)"=w180, "Right axis value"=0.5 ("Motor Output"), "Left axis value"=0.5 ("Motor Output"), "RobotDriveDevRef"=w181) -> ()  [unwired: 5 in, 3 out]
                }
              }
              frame #4 {
                w190 = 0.0 ("Motor Output")
                n108 = call <vilib>:"WPI_RobotDriveRefNum Registry Get.vi"("refnum name"="chasis") -> ("error out"=w188:errorcluster, "RobotDriveDevRef"=w189:T13)  [unwired: 9 in]
                n109 = call <vilib>:"WPI_RobotDriveTankDrive.vi"("error in (no error)"=w188, "Right axis value"=w190, "Left axis value"=w190, "RobotDriveDevRef"=w189) -> ()  [unwired: 5 in, 3 out]
              }
              frame #5 {
              }
            }
          }
          frame 5 {
            n110 = flat-sequence {
              tunnel: [6.0] -> w194
              tunnel: [TRUE] -> w193
              frame #0 {
                n111 = call <vilib>:"WPI_MotorControlRefNum Registry Get.vi"("refnum name"="ruedas") -> ("error out"=w195:errorcluster, "MotorControlDevRef"=w196:T6)  [unwired: 9 in]
                n112 = call <vilib>:"Spark MAX Set Sensor Position.vi"("error in"=w195, "Position"=0.0, "MotorControlDeviceRef"=w196) -> ()  [unwired: 7 in, 2 out]
              }
              frame #1 {
                n113 = while {
                  stop <- w203 stop-if-true
                  # "gira izquierda"
                  n114 = global read "Robot Global Data.vi" "ruedader"() -> (w205:dbl)
                  n115 = call <vilib>:"WPI_RobotDriveRefNum Registry Get.vi"("refnum name"="chasis") -> ("error out"=w199:errorcluster, "RobotDriveDevRef"=w200:T13)  [unwired: 9 in]
                  n116 = Greater Or Equal?(x=w205, y=20.0) -> (x >= y?=w203:bool)
                  n117 = call <vilib>:"WPI_RobotDriveTankDrive.vi"("error in (no error)"=w199, "Right axis value"=-0.5 ("Motor Output"), "Left axis value"=0.5 ("Motor Output"), "RobotDriveDevRef"=w200) -> ()  [unwired: 5 in, 3 out]
                }
              }
              frame #2 {
                n118 = call <vilib>:"WPI_MotorControlRefNum Registry Get.vi"("refnum name"="ruedas") -> ("error out"=w207:errorcluster, "MotorControlDevRef"=w208:T6)  [unwired: 9 in]
                n119 = call <vilib>:"Spark MAX Set Sensor Position.vi"("error in"=w207, "Position"=0.0, "MotorControlDeviceRef"=w208) -> ()  [unwired: 7 in, 2 out]
              }
              frame #3 {
                n120 = while {
                  stop <- w215 stop-if-true
                  # "avanza"
                  n121 = global read "Robot Global Data.vi" "ruedaiz"() -> (w217:dbl)
                  n122 = call <vilib>:"WPI_RobotDriveRefNum Registry Get.vi"("refnum name"="chasis") -> ("error out"=w211:errorcluster, "RobotDriveDevRef"=w212:T13)  [unwired: 9 in]
                  n123 = Greater Or Equal?(x=w217, y=50.0) -> (x >= y?=w215:bool)
                  n124 = call <vilib>:"WPI_RobotDriveTankDrive.vi"("error in (no error)"=w211, "Right axis value"=0.5 ("Motor Output"), "Left axis value"=0.5 ("Motor Output"), "RobotDriveDevRef"=w212) -> ()  [unwired: 5 in, 3 out]
                }
              }
              frame #4 {
                w221 = 0.0 ("Motor Output")
                n125 = call <vilib>:"WPI_RobotDriveRefNum Registry Get.vi"("refnum name"="chasis") -> ("error out"=w219:errorcluster, "RobotDriveDevRef"=w220:T13)  [unwired: 9 in]
                n126 = call <vilib>:"WPI_RobotDriveTankDrive.vi"("error in (no error)"=w219, "Right axis value"=w221, "Left axis value"=w221, "RobotDriveDevRef"=w220) -> ()  [unwired: 5 in, 3 out]
              }
              frame #5 {
              }
            }
          }
        }
      }
    }
    frame "caso2-pos2" {
      # "Colocar la garra, dejar la pieza, giro y avanzo, posiciono la garra, tomo la segunda pieza, reojo la garra, giras, avanzas, posicionas la garra, dejas la pieza"
      n127 = while {
        shift-right: [w227] -> _
        shift-left: 1.0 -> [w228]
        stop <- w226 stop-if-true
        n128 = case shown="3" w228 {
          tunnel: [1.0 w230 w263 w292 w322 w352 w382 w415 w444 w474 w504 w534 w568] -> w227
          tunnel: [_ _ _ _ _ _ _ _ _ _ _ _ w567] -> w226
          frame 0, Default {
          }
          frame 1 {
            n129 = flat-sequence {
              tunnel: [2.0] -> w230
              frame #0 {
                n130 = call <vilib>:"WPI_MotorControlRefNum Registry Get.vi"("refnum name"="bomberos") -> ("error out"=w233:errorcluster, "MotorControlDevRef"=w234:T6)  [unwired: 9 in]
                n131 = call <vilib>:"WPI_MotorControlRefNum Registry Get.vi"("refnum name"="polea") -> ("error out"=w236:errorcluster, "MotorControlDevRef"=w237:T6)  [unwired: 9 in]
                n132 = call <vilib>:"Spark MAX Set Sensor Position.vi"("error in"=w233, "Position"=0.0, "MotorControlDeviceRef"=w234) -> ()  [unwired: 7 in, 2 out]
                n133 = call <vilib>:"Spark MAX Set Sensor Position.vi"("error in"=w236, "Position"=0.0, "MotorControlDeviceRef"=w237) -> ()  [unwired: 7 in, 2 out]
              }
              frame #1 {
                n134 = while {
                  stop <- w251 stop-if-true
                  n135 = call <vilib>:"WPI_MotorControlRefNum Registry Get.vi"("refnum name"="bomberos") -> ("error out"=w240:errorcluster, "MotorControlDevRef"=w241:T6)  [unwired: 9 in]
                  n136 = global read "Robot Global Data.vi" "bomberos"() -> (w250:dbl)
                  n137 = call <vilib>:"WPI_MotorControlRefNum Registry Get.vi"("refnum name"="polea") -> ("error out"=w248:errorcluster, "MotorControlDevRef"=w243:T6)  [unwired: 9 in]
                  n138 = global read "Robot Global Data.vi" "vpolea"() -> (w253:dbl)
                  n139 = Greater Or Equal?(x=w253, y=15.0) -> (x >= y?=w245:bool)
                  n140 = Greater Or Equal?(x=w250, y=15.0) -> (x >= y?=w244:bool)
                  n141 = call <vilib>:"WPI_MotorControlSetOutput.vi"("error in (no error)"=w248, "Output"=0.5, "MotorControlDevRef"=w243) -> ()  [unwired: 6 in, 3 out]
                  n142 = And(x=w245, y=w244) -> (x .and. y?=w251:bool)
                  n143 = call <vilib>:"WPI_MotorControlSetOutput.vi"("error in (no error)"=w240, "Output"=0.5, "MotorControlDevRef"=w241) -> ()  [unwired: 6 in, 3 out]
                }
              }
              frame #2 {
                n144 = call <vilib>:"WPI_MotorControlRefNum Registry Get.vi"("refnum name"="bomberos") -> ("error out"=w256:errorcluster, "MotorControlDevRef"=w257:T6)  [unwired: 9 in]
                n145 = call <vilib>:"WPI_MotorControlRefNum Registry Get.vi"("refnum name"="polea") -> ("error out"=w259:errorcluster, "MotorControlDevRef"=w260:T6)  [unwired: 9 in]
                n146 = call <vilib>:"Spark MAX Set Sensor Position.vi"("error in"=w256, "Position"=0.0, "MotorControlDeviceRef"=w257) -> ()  [unwired: 7 in, 2 out]
                n147 = call <vilib>:"Spark MAX Set Sensor Position.vi"("error in"=w259, "Position"=0.0, "MotorControlDeviceRef"=w260) -> ()  [unwired: 7 in, 2 out]
              }
              frame #3 {
              }
            }
          }
          frame 2 {
            n148 = flat-sequence {
              tunnel: [3.0] -> w263
              frame #0 {
                n149 = call <vilib>:"WPI_SolenoidRefNum Registry Get.vi"("refnum name"="pickup") -> ("SolenoidDevRef"=w264:T11)  [unwired: 9 in, 1 out]
                n150 = call-poly <vilib>:"WPI_SolenoidSet.vi"("Value"=WPI_SolenoidValue."Reverse", "SolenoidDevRef"=w264) -> ()  [unwired: 8 in, 2 out]
                n151 = Wait (ms)(milliseconds to wait=u32 200) -> ()  [unwired: 1 out]
              }
              frame #1 {
                n152 = while {
                  stop <- w280 stop-if-true
                  n153 = call <vilib>:"WPI_MotorControlRefNum Registry Get.vi"("refnum name"="bomberos") -> ("error out"=w269:errorcluster, "MotorControlDevRef"=w270:T6)  [unwired: 9 in]
                  n154 = global read "Robot Global Data.vi" "bomberos"() -> (w279:dbl)
                  n155 = call <vilib>:"WPI_MotorControlRefNum Registry Get.vi"("refnum name"="polea") -> ("error out"=w272:errorcluster, "MotorControlDevRef"=w273:T6)  [unwired: 9 in]
                  n156 = global read "Robot Global Data.vi" "vpolea"() -> (w282:dbl)
                  n157 = Greater Or Equal?(x=w282, y=-15.0) -> (x >= y?=w275:bool)
                  n158 = Greater Or Equal?(x=w279, y=-15.0) -> (x >= y?=w274:bool)
                  n159 = And(x=w275, y=w274) -> (x .and. y?=w280:bool)
                  n160 = call <vilib>:"WPI_MotorControlSetOutput.vi"("error in (no error)"=w272, "Output"=-0.5, "MotorControlDevRef"=w273) -> ()  [unwired: 6 in, 3 out]
                  n161 = call <vilib>:"WPI_MotorControlSetOutput.vi"("error in (no error)"=w269, "Output"=-0.5, "MotorControlDevRef"=w270) -> ()  [unwired: 6 in, 3 out]
                }
              }
              frame #2 {
                n162 = call <vilib>:"WPI_MotorControlRefNum Registry Get.vi"("refnum name"="bomberos") -> ("error out"=w285:errorcluster, "MotorControlDevRef"=w286:T6)  [unwired: 9 in]
                n163 = call <vilib>:"WPI_MotorControlRefNum Registry Get.vi"("refnum name"="polea") -> ("error out"=w288:errorcluster, "MotorControlDevRef"=w289:T6)  [unwired: 9 in]
                n164 = call <vilib>:"Spark MAX Set Sensor Position.vi"("error in"=w285, "Position"=0.0, "MotorControlDeviceRef"=w286) -> ()  [unwired: 7 in, 2 out]
                n165 = call <vilib>:"Spark MAX Set Sensor Position.vi"("error in"=w288, "Position"=0.0, "MotorControlDeviceRef"=w289) -> ()  [unwired: 7 in, 2 out]
              }
              frame #3 {
              }
            }
          }
          frame 3 {
            n166 = flat-sequence {
              tunnel: [4.0] -> w292
              frame #0 {
                n167 = call <vilib>:"WPI_MotorControlRefNum Registry Get.vi"("refnum name"="ruedas") -> ("error out"=w293:errorcluster, "MotorControlDevRef"=w294:T6)  [unwired: 9 in]
                n168 = call <vilib>:"Spark MAX Set Sensor Position.vi"("error in"=w293, "Position"=0.0, "MotorControlDeviceRef"=w294) -> ()  [unwired: 7 in, 2 out]
              }
              frame #1 {
                n169 = while {
                  stop <- w301 stop-if-true
                  # "gira"
                  n170 = global read "Robot Global Data.vi" "ruedader"() -> (w303:dbl)
                  n171 = call <vilib>:"WPI_RobotDriveRefNum Registry Get.vi"("refnum name"="chasis") -> ("error out"=w297:errorcluster, "RobotDriveDevRef"=w298:T13)  [unwired: 9 in]
                  n172 = Greater Or Equal?(x=w303, y=40.0) -> (x >= y?=w301:bool)
                  n173 = call-poly <vilib>:"WPI_RobotDriveArcadeDrive.vi"("error in (no error)"=w297, "Y axis value"=-0.5 ("Motor Output"), "X axis value"=0.5 ("Motor Output"), "RobotDriveDevRef"=w298) -> ()  [unwired: 5 in, 3 out]
                }
              }
              frame #2 {
                n174 = call <vilib>:"WPI_MotorControlRefNum Registry Get.vi"("refnum name"="ruedas") -> ("error out"=w305:errorcluster, "MotorControlDevRef"=w306:T6)  [unwired: 9 in]
                n175 = call <vilib>:"Spark MAX Set Sensor Position.vi"("error in"=w305, "Position"=0.0, "MotorControlDeviceRef"=w306) -> ()  [unwired: 7 in, 2 out]
              }
              frame #3 {
                n176 = while {
                  stop <- w313 stop-if-true
                  # "avanza"
                  n177 = global read "Robot Global Data.vi" "ruedaiz"() -> (w315:dbl)
                  n178 = call <vilib>:"WPI_RobotDriveRefNum Registry Get.vi"("refnum name"="chasis") -> ("error out"=w309:errorcluster, "RobotDriveDevRef"=w310:T13)  [unwired: 9 in]
                  n179 = Greater Or Equal?(x=w315, y=50.0) -> (x >= y?=w313:bool)
                  n180 = call-poly <vilib>:"WPI_RobotDriveArcadeDrive.vi"("error in (no error)"=w309, "Y axis value"=0.5 ("Motor Output"), "X axis value"=0.5 ("Motor Output"), "RobotDriveDevRef"=w310) -> ()  [unwired: 5 in, 3 out]
                }
              }
              frame #4 {
                w319 = 0.0 ("Motor Output")
                n181 = call <vilib>:"WPI_RobotDriveRefNum Registry Get.vi"("refnum name"="chasis") -> ("error out"=w317:errorcluster, "RobotDriveDevRef"=w318:T13)  [unwired: 9 in]
                n182 = call-poly <vilib>:"WPI_RobotDriveArcadeDrive.vi"("error in (no error)"=w317, "Y axis value"=w319, "X axis value"=w319, "RobotDriveDevRef"=w318) -> ()  [unwired: 5 in, 3 out]
              }
              frame #5 {
              }
            }
          }
          frame 4 {
            n183 = flat-sequence {
              tunnel: [5.0] -> w322
              frame #0 {
                n184 = call <vilib>:"WPI_MotorControlRefNum Registry Get.vi"("refnum name"="ruedas") -> ("error out"=w323:errorcluster, "MotorControlDevRef"=w324:T6)  [unwired: 9 in]
                n185 = call <vilib>:"Spark MAX Set Sensor Position.vi"("error in"=w323, "Position"=0.0, "MotorControlDeviceRef"=w324) -> ()  [unwired: 7 in, 2 out]
              }
              frame #1 {
                n186 = while {
                  stop <- w331 stop-if-true
                  # "gira derecha"
                  n187 = global read "Robot Global Data.vi" "ruedader"() -> (w333:dbl)
                  n188 = call <vilib>:"WPI_RobotDriveRefNum Registry Get.vi"("refnum name"="chasis") -> ("error out"=w327:errorcluster, "RobotDriveDevRef"=w328:T13)  [unwired: 9 in]
                  n189 = Greater Or Equal?(x=w333, y=20.0) -> (x >= y?=w331:bool)
                  n190 = call <vilib>:"WPI_RobotDriveTankDrive.vi"("error in (no error)"=w327, "Right axis value"=0.5 ("Motor Output"), "Left axis value"=-0.5 ("Motor Output"), "RobotDriveDevRef"=w328) -> ()  [unwired: 5 in, 3 out]
                }
              }
              frame #2 {
                n191 = call <vilib>:"WPI_MotorControlRefNum Registry Get.vi"("refnum name"="ruedas") -> ("error out"=w335:errorcluster, "MotorControlDevRef"=w336:T6)  [unwired: 9 in]
                n192 = call <vilib>:"Spark MAX Set Sensor Position.vi"("error in"=w335, "Position"=0.0, "MotorControlDeviceRef"=w336) -> ()  [unwired: 7 in, 2 out]
              }
              frame #3 {
                n193 = while {
                  stop <- w343 stop-if-true
                  # "avanza"
                  n194 = global read "Robot Global Data.vi" "ruedaiz"() -> (w345:dbl)
                  n195 = call <vilib>:"WPI_RobotDriveRefNum Registry Get.vi"("refnum name"="chasis") -> ("error out"=w339:errorcluster, "RobotDriveDevRef"=w340:T13)  [unwired: 9 in]
                  n196 = Greater Or Equal?(x=w345, y=25.0) -> (x >= y?=w343:bool)
                  n197 = call <vilib>:"WPI_RobotDriveTankDrive.vi"("error in (no error)"=w339, "Right axis value"=0.5 ("Motor Output"), "Left axis value"=0.5 ("Motor Output"), "RobotDriveDevRef"=w340) -> ()  [unwired: 5 in, 3 out]
                }
              }
              frame #4 {
                w349 = 0.0 ("Motor Output")
                n198 = call <vilib>:"WPI_RobotDriveRefNum Registry Get.vi"("refnum name"="chasis") -> ("error out"=w347:errorcluster, "RobotDriveDevRef"=w348:T13)  [unwired: 9 in]
                n199 = call <vilib>:"WPI_RobotDriveTankDrive.vi"("error in (no error)"=w347, "Right axis value"=w349, "Left axis value"=w349, "RobotDriveDevRef"=w348) -> ()  [unwired: 5 in, 3 out]
              }
              frame #5 {
              }
            }
          }
          frame 5 {
            n200 = flat-sequence {
              tunnel: [6.0] -> w352
              frame #0 {
                n201 = call <vilib>:"WPI_MotorControlRefNum Registry Get.vi"("refnum name"="ruedas") -> ("error out"=w353:errorcluster, "MotorControlDevRef"=w354:T6)  [unwired: 9 in]
                n202 = call <vilib>:"Spark MAX Set Sensor Position.vi"("error in"=w353, "Position"=0.0, "MotorControlDeviceRef"=w354) -> ()  [unwired: 7 in, 2 out]
              }
              frame #1 {
                n203 = while {
                  stop <- w361 stop-if-true
                  # "gira izquierda"
                  n204 = global read "Robot Global Data.vi" "ruedader"() -> (w363:dbl)
                  n205 = call <vilib>:"WPI_RobotDriveRefNum Registry Get.vi"("refnum name"="chasis") -> ("error out"=w357:errorcluster, "RobotDriveDevRef"=w358:T13)  [unwired: 9 in]
                  n206 = Greater Or Equal?(x=w363, y=20.0) -> (x >= y?=w361:bool)
                  n207 = call <vilib>:"WPI_RobotDriveTankDrive.vi"("error in (no error)"=w357, "Right axis value"=-0.5 ("Motor Output"), "Left axis value"=0.5 ("Motor Output"), "RobotDriveDevRef"=w358) -> ()  [unwired: 5 in, 3 out]
                }
              }
              frame #2 {
                n208 = call <vilib>:"WPI_MotorControlRefNum Registry Get.vi"("refnum name"="ruedas") -> ("error out"=w365:errorcluster, "MotorControlDevRef"=w366:T6)  [unwired: 9 in]
                n209 = call <vilib>:"Spark MAX Set Sensor Position.vi"("error in"=w365, "Position"=0.0, "MotorControlDeviceRef"=w366) -> ()  [unwired: 7 in, 2 out]
              }
              frame #3 {
                n210 = while {
                  stop <- w373 stop-if-true
                  # "avanza"
                  n211 = global read "Robot Global Data.vi" "ruedaiz"() -> (w375:dbl)
                  n212 = call <vilib>:"WPI_RobotDriveRefNum Registry Get.vi"("refnum name"="chasis") -> ("error out"=w369:errorcluster, "RobotDriveDevRef"=w370:T13)  [unwired: 9 in]
                  n213 = Greater Or Equal?(x=w375, y=50.0) -> (x >= y?=w373:bool)
                  n214 = call <vilib>:"WPI_RobotDriveTankDrive.vi"("error in (no error)"=w369, "Right axis value"=0.5 ("Motor Output"), "Left axis value"=0.5 ("Motor Output"), "RobotDriveDevRef"=w370) -> ()  [unwired: 5 in, 3 out]
                }
              }
              frame #4 {
                w379 = 0.0 ("Motor Output")
                n215 = call <vilib>:"WPI_RobotDriveRefNum Registry Get.vi"("refnum name"="chasis") -> ("error out"=w377:errorcluster, "RobotDriveDevRef"=w378:T13)  [unwired: 9 in]
                n216 = call <vilib>:"WPI_RobotDriveTankDrive.vi"("error in (no error)"=w377, "Right axis value"=w379, "Left axis value"=w379, "RobotDriveDevRef"=w378) -> ()  [unwired: 5 in, 3 out]
              }
              frame #5 {
              }
            }
          }
          frame 6 {
            n217 = flat-sequence {
              tunnel: [7.0] -> w382
              frame #0 {
                n218 = call <vilib>:"WPI_MotorControlRefNum Registry Get.vi"("refnum name"="polea") -> ("error out"=w383:errorcluster, "MotorControlDevRef"=w384:T6)  [unwired: 9 in]
                n219 = call <vilib>:"Spark MAX Set Sensor Position.vi"("error in"=w383, "Position"=0.0, "MotorControlDeviceRef"=w384) -> ()  [unwired: 7 in, 2 out]
                n220 = call <vilib>:"WPI_MotorControlRefNum Registry Get.vi"("refnum name"="bomberos") -> ("error out"=w387:errorcluster, "MotorControlDevRef"=w388:T6)  [unwired: 9 in]
                n221 = call <vilib>:"Spark MAX Set Sensor Position.vi"("error in"=w387, "Position"=0.0, "MotorControlDeviceRef"=w388) -> ()  [unwired: 7 in, 2 out]
              }
              frame #1 {
                n222 = while {
                  stop <- w395 stop-if-true
                  n223 = global read "Robot Global Data.vi" "bomberos"() -> (w397:dbl)
                  n224 = call <vilib>:"WPI_MotorControlRefNum Registry Get.vi"("refnum name"="bomberos") -> ("error out"=w405:errorcluster, "MotorControlDevRef"=w404:T6)  [unwired: 9 in]
                  n225 = global read "Robot Global Data.vi" "vpolea"() -> (w393:dbl)
                  n226 = call <vilib>:"WPI_MotorControlSetOutput.vi"("error in (no error)"=w405, "Output"=-0.5 ("Motor Output"), "MotorControlDevRef"=w404) -> ()  [unwired: 6 in, 3 out]
                  n227 = Greater Or Equal?(x=w397, y=20.0) -> (x >= y?=w396:bool)
                  n228 = Greater Or Equal?(x=w393, y=20.0) -> (x >= y?=w391:bool)
                  n229 = call <vilib>:"WPI_MotorControlRefNum Registry Get.vi"("refnum name"="polea") -> ("error out"=w401:errorcluster, "MotorControlDevRef"=w400:T6)  [unwired: 9 in]
                  n230 = And(x=w396, y=w391) -> (x .and. y?=w395:bool)
                  n231 = call <vilib>:"WPI_MotorControlSetOutput.vi"("error in (no error)"=w401, "Output"=0.5 ("Motor Output"), "MotorControlDevRef"=w400) -> ()  [unwired: 6 in, 3 out]
                }
              }
              frame #2 {
                n232 = call <vilib>:"WPI_MotorControlRefNum Registry Get.vi"("refnum name"="polea") -> ("error out"=w412:errorcluster, "MotorControlDevRef"=w413:T6)  [unwired: 9 in]
                n233 = call <vilib>:"WPI_MotorControlRefNum Registry Get.vi"("refnum name"="bomberos") -> ("error out"=w410:errorcluster, "MotorControlDevRef"=w411:T6)  [unwired: 9 in]
                n234 = call <vilib>:"WPI_MotorControlSetOutput.vi"("error in (no error)"=w412, "Output"=0.0 ("Motor Output"), "MotorControlDevRef"=w413) -> ()  [unwired: 6 in, 3 out]
                n235 = call <vilib>:"WPI_MotorControlSetOutput.vi"("error in (no error)"=w410, "Output"=0.0 ("Motor Output"), "MotorControlDevRef"=w411) -> ()  [unwired: 6 in, 3 out]
              }
              frame #3 {
              }
            }
          }
          frame 7 {
            n236 = flat-sequence {
              tunnel: [8.0] -> w415
              frame #0 {
                n237 = Wait (ms)(milliseconds to wait=u32 200) -> ()  [unwired: 1 out]
                n238 = call <vilib>:"WPI_SolenoidRefNum Registry Get.vi"("refnum name"="pickup") -> ("SolenoidDevRef"=w419:T11)  [unwired: 9 in, 1 out]
                n239 = call-poly <vilib>:"WPI_SolenoidSet.vi"("Value"=WPI_SolenoidValue."Forward", "SolenoidDevRef"=w419) -> ()  [unwired: 8 in, 2 out]
              }
              frame #1 {
                n240 = while {
                  stop <- w432 stop-if-true
                  n241 = call <vilib>:"WPI_MotorControlRefNum Registry Get.vi"("refnum name"="bomberos") -> ("error out"=w421:errorcluster, "MotorControlDevRef"=w422:T6)  [unwired: 9 in]
                  n242 = global read "Robot Global Data.vi" "bomberos"() -> (w431:dbl)
                  n243 = call <vilib>:"WPI_MotorControlRefNum Registry Get.vi"("refnum name"="polea") -> ("error out"=w424:errorcluster, "MotorControlDevRef"=w425:T6)  [unwired: 9 in]
                  n244 = global read "Robot Global Data.vi" "vpolea"() -> (w434:dbl)
                  n245 = Greater Or Equal?(x=w434, y=15.0) -> (x >= y?=w427:bool)
                  n246 = Greater Or Equal?(x=w431, y=15.0) -> (x >= y?=w426:bool)
                  n247 = call <vilib>:"WPI_MotorControlSetOutput.vi"("error in (no error)"=w421, "Output"=-0.5, "MotorControlDevRef"=w422) -> ()  [unwired: 6 in, 3 out]
                  n248 = And(x=w427, y=w426) -> (x .and. y?=w432:bool)
                  n249 = call <vilib>:"WPI_MotorControlSetOutput.vi"("error in (no error)"=w424, "Output"=0.5, "MotorControlDevRef"=w425) -> ()  [unwired: 6 in, 3 out]
                }
              }
              frame #2 {
                n250 = call <vilib>:"WPI_MotorControlRefNum Registry Get.vi"("refnum name"="bomberos") -> ("error out"=w437:errorcluster, "MotorControlDevRef"=w438:T6)  [unwired: 9 in]
                n251 = call <vilib>:"WPI_MotorControlRefNum Registry Get.vi"("refnum name"="polea") -> ("error out"=w440:errorcluster, "MotorControlDevRef"=w441:T6)  [unwired: 9 in]
                n252 = call <vilib>:"Spark MAX Set Sensor Position.vi"("error in"=w437, "Position"=0.0, "MotorControlDeviceRef"=w438) -> ()  [unwired: 7 in, 2 out]
                n253 = call <vilib>:"Spark MAX Set Sensor Position.vi"("error in"=w440, "Position"=0.0, "MotorControlDeviceRef"=w441) -> ()  [unwired: 7 in, 2 out]
              }
              frame #3 {
              }
            }
          }
          frame 8 {
            n254 = flat-sequence {
              tunnel: [9.0] -> w444
              frame #0 {
                n255 = call <vilib>:"WPI_MotorControlRefNum Registry Get.vi"("refnum name"="ruedas") -> ("error out"=w445:errorcluster, "MotorControlDevRef"=w446:T6)  [unwired: 9 in]
                n256 = call <vilib>:"Spark MAX Set Sensor Position.vi"("error in"=w445, "Position"=0.0, "MotorControlDeviceRef"=w446) -> ()  [unwired: 7 in, 2 out]
              }
              frame #1 {
                n257 = while {
                  stop <- w453 stop-if-true
                  # "gira"
                  n258 = global read "Robot Global Data.vi" "ruedaiz"() -> (w455:dbl)
                  n259 = call <vilib>:"WPI_RobotDriveRefNum Registry Get.vi"("refnum name"="chasis") -> ("error out"=w449:errorcluster, "RobotDriveDevRef"=w450:T13)  [unwired: 9 in]
                  n260 = Greater Or Equal?(x=w455, y=40.0) -> (x >= y?=w453:bool)
                  n261 = call <vilib>:"WPI_RobotDriveTankDrive.vi"("error in (no error)"=w449, "Right axis value"=-0.5 ("Motor Output"), "Left axis value"=0.5 ("Motor Output"), "RobotDriveDevRef"=w450) -> ()  [unwired: 5 in, 3 out]
                }
              }
              frame #2 {
                n262 = call <vilib>:"WPI_MotorControlRefNum Registry Get.vi"("refnum name"="ruedas") -> ("error out"=w457:errorcluster, "MotorControlDevRef"=w458:T6)  [unwired: 9 in]
                n263 = call <vilib>:"Spark MAX Set Sensor Position.vi"("error in"=w457, "Position"=0.0, "MotorControlDeviceRef"=w458) -> ()  [unwired: 7 in, 2 out]
              }
              frame #3 {
                n264 = while {
                  stop <- w465 stop-if-true
                  # "avanza"
                  n265 = global read "Robot Global Data.vi" "ruedader"() -> (w467:dbl)
                  n266 = call <vilib>:"WPI_RobotDriveRefNum Registry Get.vi"("refnum name"="chasis") -> ("error out"=w461:errorcluster, "RobotDriveDevRef"=w462:T13)  [unwired: 9 in]
                  n267 = Greater Or Equal?(x=w467, y=75.0) -> (x >= y?=w465:bool)
                  n268 = call <vilib>:"WPI_RobotDriveTankDrive.vi"("error in (no error)"=w461, "Right axis value"=0.5 ("Motor Output"), "Left axis value"=0.5 ("Motor Output"), "RobotDriveDevRef"=w462) -> ()  [unwired: 5 in, 3 out]
                }
              }
              frame #4 {
                w471 = 0.0 ("Motor Output")
                n269 = call <vilib>:"WPI_RobotDriveRefNum Registry Get.vi"("refnum name"="chasis") -> ("error out"=w469:errorcluster, "RobotDriveDevRef"=w470:T13)  [unwired: 9 in]
                n270 = call <vilib>:"WPI_RobotDriveTankDrive.vi"("error in (no error)"=w469, "Right axis value"=w471, "Left axis value"=w471, "RobotDriveDevRef"=w470) -> ()  [unwired: 5 in, 3 out]
              }
              frame #5 {
              }
            }
          }
          frame 9 {
            n271 = flat-sequence {
              tunnel: [10.0] -> w474
              frame #0 {
                n272 = call <vilib>:"WPI_MotorControlRefNum Registry Get.vi"("refnum name"="ruedas") -> ("error out"=w475:errorcluster, "MotorControlDevRef"=w476:T6)  [unwired: 9 in]
                n273 = call <vilib>:"Spark MAX Set Sensor Position.vi"("error in"=w475, "Position"=0.0, "MotorControlDeviceRef"=w476) -> ()  [unwired: 7 in, 2 out]
              }
              frame #1 {
                n274 = while {
                  stop <- w483 stop-if-true
                  # "gira derecha"
                  n275 = global read "Robot Global Data.vi" "ruedader"() -> (w485:dbl)
                  n276 = call <vilib>:"WPI_RobotDriveRefNum Registry Get.vi"("refnum name"="chasis") -> ("error out"=w479:errorcluster, "RobotDriveDevRef"=w480:T13)  [unwired: 9 in]
                  n277 = Greater Or Equal?(x=w485, y=20.0) -> (x >= y?=w483:bool)
                  n278 = call <vilib>:"WPI_RobotDriveTankDrive.vi"("error in (no error)"=w479, "Right axis value"=0.5 ("Motor Output"), "Left axis value"=-0.5 ("Motor Output"), "RobotDriveDevRef"=w480) -> ()  [unwired: 5 in, 3 out]
                }
              }
              frame #2 {
                n279 = call <vilib>:"WPI_MotorControlRefNum Registry Get.vi"("refnum name"="ruedas") -> ("error out"=w487:errorcluster, "MotorControlDevRef"=w488:T6)  [unwired: 9 in]
                n280 = call <vilib>:"Spark MAX Set Sensor Position.vi"("error in"=w487, "Position"=0.0, "MotorControlDeviceRef"=w488) -> ()  [unwired: 7 in, 2 out]
              }
              frame #3 {
                n281 = while {
                  stop <- w495 stop-if-true
                  # "avanza"
                  n282 = global read "Robot Global Data.vi" "ruedaiz"() -> (w497:dbl)
                  n283 = call <vilib>:"WPI_RobotDriveRefNum Registry Get.vi"("refnum name"="chasis") -> ("error out"=w491:errorcluster, "RobotDriveDevRef"=w492:T13)  [unwired: 9 in]
                  n284 = Greater Or Equal?(x=w497, y=25.0) -> (x >= y?=w495:bool)
                  n285 = call <vilib>:"WPI_RobotDriveTankDrive.vi"("error in (no error)"=w491, "Right axis value"=0.5 ("Motor Output"), "Left axis value"=0.5 ("Motor Output"), "RobotDriveDevRef"=w492) -> ()  [unwired: 5 in, 3 out]
                }
              }
              frame #4 {
                w501 = 0.0 ("Motor Output")
                n286 = call <vilib>:"WPI_RobotDriveRefNum Registry Get.vi"("refnum name"="chasis") -> ("error out"=w499:errorcluster, "RobotDriveDevRef"=w500:T13)  [unwired: 9 in]
                n287 = call <vilib>:"WPI_RobotDriveTankDrive.vi"("error in (no error)"=w499, "Right axis value"=w501, "Left axis value"=w501, "RobotDriveDevRef"=w500) -> ()  [unwired: 5 in, 3 out]
              }
              frame #5 {
              }
            }
          }
          frame 10 {
            n288 = flat-sequence {
              tunnel: [11.0] -> w504
              frame #0 {
                n289 = call <vilib>:"WPI_MotorControlRefNum Registry Get.vi"("refnum name"="ruedas") -> ("error out"=w505:errorcluster, "MotorControlDevRef"=w506:T6)  [unwired: 9 in]
                n290 = call <vilib>:"Spark MAX Set Sensor Position.vi"("error in"=w505, "Position"=0.0, "MotorControlDeviceRef"=w506) -> ()  [unwired: 7 in, 2 out]
              }
              frame #1 {
                n291 = while {
                  stop <- w513 stop-if-true
                  # "gira izquierda"
                  n292 = global read "Robot Global Data.vi" "ruedader"() -> (w515:dbl)
                  n293 = call <vilib>:"WPI_RobotDriveRefNum Registry Get.vi"("refnum name"="chasis") -> ("error out"=w509:errorcluster, "RobotDriveDevRef"=w510:T13)  [unwired: 9 in]
                  n294 = Greater Or Equal?(x=w515, y=20.0) -> (x >= y?=w513:bool)
                  n295 = call <vilib>:"WPI_RobotDriveTankDrive.vi"("error in (no error)"=w509, "Right axis value"=-0.5 ("Motor Output"), "Left axis value"=0.5 ("Motor Output"), "RobotDriveDevRef"=w510) -> ()  [unwired: 5 in, 3 out]
                }
              }
              frame #2 {
                n296 = call <vilib>:"WPI_MotorControlRefNum Registry Get.vi"("refnum name"="ruedas") -> ("error out"=w517:errorcluster, "MotorControlDevRef"=w518:T6)  [unwired: 9 in]
                n297 = call <vilib>:"Spark MAX Set Sensor Position.vi"("error in"=w517, "Position"=0.0, "MotorControlDeviceRef"=w518) -> ()  [unwired: 7 in, 2 out]
              }
              frame #3 {
                n298 = while {
                  stop <- w525 stop-if-true
                  # "avanza"
                  n299 = global read "Robot Global Data.vi" "ruedaiz"() -> (w527:dbl)
                  n300 = call <vilib>:"WPI_RobotDriveRefNum Registry Get.vi"("refnum name"="chasis") -> ("error out"=w521:errorcluster, "RobotDriveDevRef"=w522:T13)  [unwired: 9 in]
                  n301 = Greater Or Equal?(x=w527, y=50.0) -> (x >= y?=w525:bool)
                  n302 = call <vilib>:"WPI_RobotDriveTankDrive.vi"("error in (no error)"=w521, "Right axis value"=0.5 ("Motor Output"), "Left axis value"=0.5 ("Motor Output"), "RobotDriveDevRef"=w522) -> ()  [unwired: 5 in, 3 out]
                }
              }
              frame #4 {
                w531 = 0.0 ("Motor Output")
                n303 = call <vilib>:"WPI_RobotDriveRefNum Registry Get.vi"("refnum name"="chasis") -> ("error out"=w529:errorcluster, "RobotDriveDevRef"=w530:T13)  [unwired: 9 in]
                n304 = call <vilib>:"WPI_RobotDriveTankDrive.vi"("error in (no error)"=w529, "Right axis value"=w531, "Left axis value"=w531, "RobotDriveDevRef"=w530) -> ()  [unwired: 5 in, 3 out]
              }
              frame #5 {
              }
            }
          }
          frame 11 {
            n305 = flat-sequence {
              tunnel: [12.0] -> w534
              frame #0 {
                n306 = call <vilib>:"WPI_MotorControlRefNum Registry Get.vi"("refnum name"="bomberos") -> ("error out"=w537:errorcluster, "MotorControlDevRef"=w538:T6)  [unwired: 9 in]
                n307 = call <vilib>:"WPI_MotorControlRefNum Registry Get.vi"("refnum name"="polea") -> ("error out"=w540:errorcluster, "MotorControlDevRef"=w541:T6)  [unwired: 9 in]
                n308 = call <vilib>:"Spark MAX Set Sensor Position.vi"("error in"=w537, "Position"=0.0, "MotorControlDeviceRef"=w538) -> ()  [unwired: 7 in, 2 out]
                n309 = call <vilib>:"Spark MAX Set Sensor Position.vi"("error in"=w540, "Position"=0.0, "MotorControlDeviceRef"=w541) -> ()  [unwired: 7 in, 2 out]
              }
              frame #1 {
                n310 = while {
                  stop <- w555 stop-if-true
                  n311 = call <vilib>:"WPI_MotorControlRefNum Registry Get.vi"("refnum name"="bomberos") -> ("error out"=w544:errorcluster, "MotorControlDevRef"=w545:T6)  [unwired: 9 in]
                  n312 = global read "Robot Global Data.vi" "bomberos"() -> (w554:dbl)
                  n313 = call <vilib>:"WPI_MotorControlRefNum Registry Get.vi"("refnum name"="polea") -> ("error out"=w547:errorcluster, "MotorControlDevRef"=w548:T6)  [unwired: 9 in]
                  n314 = global read "Robot Global Data.vi" "vpolea"() -> (w557:dbl)
                  n315 = Greater Or Equal?(x=w557, y=15.0) -> (x >= y?=w550:bool)
                  n316 = Greater Or Equal?(x=w554, y=15.0) -> (x >= y?=w549:bool)
                  n317 = And(x=w550, y=w549) -> (x .and. y?=w555:bool)
                  n318 = call <vilib>:"WPI_MotorControlSetOutput.vi"("error in (no error)"=w544, "Output"=0.5, "MotorControlDevRef"=w545) -> ()  [unwired: 6 in, 3 out]
                  n319 = call <vilib>:"WPI_MotorControlSetOutput.vi"("error in (no error)"=w547, "Output"=-0.5, "MotorControlDevRef"=w548) -> ()  [unwired: 6 in, 3 out]
                }
              }
              frame #2 {
                n320 = call <vilib>:"WPI_MotorControlRefNum Registry Get.vi"("refnum name"="bomberos") -> ("error out"=w560:errorcluster, "MotorControlDevRef"=w561:T6)  [unwired: 9 in]
                n321 = call <vilib>:"WPI_MotorControlRefNum Registry Get.vi"("refnum name"="polea") -> ("error out"=w563:errorcluster, "MotorControlDevRef"=w564:T6)  [unwired: 9 in]
                n322 = call <vilib>:"Spark MAX Set Sensor Position.vi"("error in"=w560, "Position"=0.0, "MotorControlDeviceRef"=w561) -> ()  [unwired: 7 in, 2 out]
                n323 = call <vilib>:"Spark MAX Set Sensor Position.vi"("error in"=w563, "Position"=0.0, "MotorControlDeviceRef"=w564) -> ()  [unwired: 7 in, 2 out]
              }
              frame #3 {
              }
            }
          }
          frame 12 {
            n324 = flat-sequence {
              tunnel: [13.0] -> w568
              tunnel: [TRUE] -> w567
              frame #0 {
                n325 = call <vilib>:"WPI_SolenoidRefNum Registry Get.vi"("refnum name"="pickup") -> ("SolenoidDevRef"=w569:T11)  [unwired: 9 in, 1 out]
                n326 = call-poly <vilib>:"WPI_SolenoidSet.vi"("Value"=WPI_SolenoidValue."Reverse", "SolenoidDevRef"=w569) -> ()  [unwired: 8 in, 2 out]
                n327 = Wait (ms)(milliseconds to wait=u32 200) -> ()  [unwired: 1 out]
              }
              frame #1 {
              }
            }
          }
        }
      }
    }
    frame "Alternative 1" {
      # "stand still"
      # "This sample code describes robot movements in an array. You can extend it to control other motors\non your robot. You can also use file I/O to move the data to a text file."
      n328 = call <vilib>:"WPI_RobotDriveRefNum Registry Get.vi"("refnum name"="Left and Right Motors") -> ("RobotDriveDevRef"=w581:T13)  [unwired: 1 in, 9 out]
      n329 = for {
        shift-right: [w589] -> w576
        shift-left: w581 -> [w590]
        tunnel: "Array of robot movements" -> [w585] mode=indexing
        n330 = Unbundle By Name(w585) -> ("X Joystick Value"=w588:dbl, "Y Joystick Value"=w587:dbl, "Delay (sec)"=w586:dbl)  [unwired: 1 out]
        n331 = call-poly <vilib>:"WPI_RobotDriveArcadeDrive.vi"("Y axis value"=w587, "X axis value"=w588, "RobotDriveDevRef"=w590) -> ("Motor Values"=w583:dbl[], "RobotDriveDevRef"=w591:T13)  [unwired: 1 in, 6 out]
        n332 = call-poly <vilib>:"NT Write Value.vi"("Numeric Array"=w583, "Name"="RobotDrive Motors") -> ()  [unwired: 9 in, 1 out]
        n333 = call <vilib>:"WPI_RobotDriveDelayAndUpdateSafety.vi"("Delay (s)"=w586, "RobotDriveDevRef"=w591) -> ("RobotDriveDevRef 2"=w589:T13)  [unwired: 8 in, 1 out]
        "Current Movement, for debugging" <- w585
      }
      n334 = call-poly <vilib>:"WPI_RobotDriveArcadeDrive.vi"("Y axis value"=0.0 ("X axis value"), "X axis value"=0.0, "RobotDriveDevRef"=w576) -> ("Motor Values"=w579:dbl[])  [unwired: 1 in, 7 out]
      n335 = call-poly <vilib>:"NT Write Value.vi"("Numeric Array"=w579, "Name"="RobotDrive Motors") -> ()  [unwired: 9 in, 1 out]
    }
    frame "Alternative 2" {
      # "Prueba exclusiva de balanceo"
      n336 = global read "Robot Global Data.vi" "full_reverse_arduino"() -> (w597:bool)
      n337 = global read "Robot Global Data.vi" "stop_arduino"() -> (w599:bool)
      n338 = global read "Robot Global Data.vi" "full_forward_arduino"() -> (w598:bool)
      n339 = Build Array(w599, w598, w597) -> (w596:bool[])
      n340 = Boolean Array To Number(Boolean array=w596) -> (number=w593:u32)
      n341 = call <vilib>:"WPI_RobotDriveRefNum Registry Get.vi"("refnum name"="chasis") -> ("error out"=w594:errorcluster, "RobotDriveDevRef"=w595:T13)  [unwired: 9 in]
      n342 = case shown="4" w593 {
        tunnel: [0.0 0.0 0.4 -0.4] -> w592
        frame 0, Default {
        }
        frame 1 {
        }
        frame 2 {
        }
        frame 4 {
        }
      }
      n343 = call <vilib>:"WPI_RobotDriveTankDrive.vi"("error in (no error)"=w594, "Right axis value"=w592, "Left axis value"=w592, "RobotDriveDevRef"=w595) -> ()  [unwired: 5 in, 3 out]
    }
    frame "caso1-pos1-t" {
      n344 = while {
        shift-right: [w608] -> _
        shift-left: 1.0 -> [w606]
        stop <- w607 stop-if-true
        n345 = case shown="3" w606 {
          tunnel: [1.0 w610 w630 w640] -> w608
          tunnel: [_ _ _ w639] -> w607
          frame 0, Default {
          }
          frame 1 {
            n346 = flat-sequence {
              tunnel: [2.0] -> w610
              frame #0 {
                n347 = call <vilib>:"WPI_MotorControlRefNum Registry Get.vi"("refnum name"="polea") -> ("error out"=w614:errorcluster, "MotorControlDevRef"=w615:T6)  [unwired: 9 in]
                n348 = Wait (ms)(milliseconds to wait=u32 150) -> ()  [unwired: 1 out]
                n349 = call <vilib>:"WPI_MotorControlSetOutput.vi"("error in (no error)"=w614, "Output"=-0.5, "MotorControlDevRef"=w615) -> ()  [unwired: 6 in, 3 out]
              }
              frame #1 {
                n350 = call <vilib>:"WPI_MotorControlRefNum Registry Get.vi"("refnum name"="bomberos") -> ("error out"=w624:errorcluster, "MotorControlDevRef"=w623:T6)  [unwired: 9 in]
                n351 = call <vilib>:"WPI_MotorControlRefNum Registry Get.vi"("refnum name"="polea") -> ("error out"=w618:errorcluster, "MotorControlDevRef"=w619:T6)  [unwired: 9 in]
                n352 = call <vilib>:"WPI_MotorControlSetOutput.vi"("error in (no error)"=w624, "Output"=0.5, "MotorControlDevRef"=w623) -> ()  [unwired: 6 in, 3 out]
                n353 = call <vilib>:"WPI_MotorControlSetOutput.vi"("error in (no error)"=w618, "Output"=0.0, "MotorControlDevRef"=w619) -> ()  [unwired: 6 in, 3 out]
                n354 = Wait (ms)(milliseconds to wait=u32 200) -> ()  [unwired: 1 out]
              }
              frame #2 {
                n355 = call <vilib>:"WPI_MotorControlRefNum Registry Get.vi"("refnum name"="bomberos") -> ("error out"=w627:errorcluster, "MotorControlDevRef"=w628:T6)  [unwired: 9 in]
                n356 = call <vilib>:"WPI_MotorControlSetOutput.vi"("error in (no error)"=w627, "Output"=0.0, "MotorControlDevRef"=w628) -> ()  [unwired: 6 in, 3 out]
              }
              frame #3 {
              }
            }
          }
          frame 2 {
            n357 = flat-sequence {
              tunnel: [3.0] -> w630
              frame #0 {
                n358 = call <vilib>:"WPI_SolenoidRefNum Registry Get.vi"("refnum name"="pickup") -> ("SolenoidDevRef"=w633:T11)  [unwired: 9 in, 1 out]
                n359 = call-poly <vilib>:"WPI_SolenoidSet.vi"("Value"=WPI_SolenoidValue."Reverse", "SolenoidDevRef"=w633) -> ()  [unwired: 8 in, 2 out]
                n360 = Wait (ms)(milliseconds to wait=u32 200) -> ()  [unwired: 1 out]
              }
              frame #1 {
                n361 = call <vilib>:"WPI_SolenoidRefNum Registry Get.vi"("refnum name"="pickup") -> ("SolenoidDevRef"=w637:T11)  [unwired: 9 in, 1 out]
                n362 = call-poly <vilib>:"WPI_SolenoidSet.vi"("Value"=WPI_SolenoidValue."Forward", "SolenoidDevRef"=w637) -> ()  [unwired: 8 in, 2 out]
              }
              frame #2 {
              }
            }
          }
          frame 3 {
            n363 = flat-sequence {
              tunnel: [4.0] -> w640
              tunnel: [TRUE] -> w639
              frame #0 {
                n364 = call <vilib>:"WPI_RobotDriveRefNum Registry Get.vi"("refnum name"="chasis") -> ("error out"=w647:errorcluster, "RobotDriveDevRef"=w648:T13)  [unwired: 9 in]
                n365 = call <vilib>:"WPI_RobotDriveTankDrive.vi"("error in (no error)"=w647, "Right axis value"=-0.5 ("Motor Output"), "Left axis value"=0.5 ("Motor Output"), "RobotDriveDevRef"=w648) -> ("error out"=w642:errorcluster, "RobotDriveDevRef"=w643:T13)  [unwired: 5 in, 1 out]
                n366 = call <vilib>:"WPI_RobotDriveDelayAndUpdateSafety.vi"("error in (no error)"=w642, "Delay (s)"=2.0, "RobotDriveDevRef"=w643) -> ()  [unwired: 7 in, 2 out]
              }
              frame #1 {
                w649 = 0.0 ("Motor Output")
                n367 = call <vilib>:"WPI_RobotDriveRefNum Registry Get.vi"("refnum name"="chasis") -> ("error out"=w652:errorcluster, "RobotDriveDevRef"=w651:T13)  [unwired: 9 in]
                n368 = call <vilib>:"WPI_RobotDriveTankDrive.vi"("error in (no error)"=w652, "Right axis value"=w649, "Left axis value"=w649, "RobotDriveDevRef"=w651) -> ()  [unwired: 5 in, 3 out]
              }
              frame #2 {
                w656 = 0.5 ("Motor Output")
                n369 = call <vilib>:"WPI_RobotDriveRefNum Registry Get.vi"("refnum name"="chasis") -> ("error out"=w659:errorcluster, "RobotDriveDevRef"=w658:T13)  [unwired: 9 in]
                n370 = call <vilib>:"WPI_RobotDriveTankDrive.vi"("error in (no error)"=w659, "Right axis value"=w656, "Left axis value"=w656, "RobotDriveDevRef"=w658) -> ("error out"=w655:errorcluster, "RobotDriveDevRef"=w654:T13)  [unwired: 5 in, 1 out]
                n371 = call <vilib>:"WPI_RobotDriveDelayAndUpdateSafety.vi"("error in (no error)"=w655, "Delay (s)"=5.0, "RobotDriveDevRef"=w654) -> ()  [unwired: 7 in, 2 out]
              }
              frame #3 {
                w660 = 0.0 ("Motor Output")
                n372 = call <vilib>:"WPI_RobotDriveRefNum Registry Get.vi"("refnum name"="chasis") -> ("error out"=w663:errorcluster, "RobotDriveDevRef"=w662:T13)  [unwired: 9 in]
                n373 = call <vilib>:"WPI_RobotDriveTankDrive.vi"("error in (no error)"=w663, "Right axis value"=w660, "Left axis value"=w660, "RobotDriveDevRef"=w662) -> ()  [unwired: 5 in, 3 out]
              }
              frame #4 {
              }
            }
          }
        }
      }
    }
    frame "caso2-pos1-t" {
      n374 = while {
        shift-right: [w668] -> _
        shift-left: 1.0 -> [w669]
        stop <- w667 stop-if-true
        n375 = case shown="2" w669 {
          tunnel: [1.0 w671 w690 w696 w718 w737 w743 w762 w784 w804] -> w668
          tunnel: [_ _ _ _ _ _ _ _ _ w803] -> w667
          frame 0, Default {
          }
          frame 1 {
            n376 = flat-sequence {
              tunnel: [2.0] -> w671
              frame #0 {
                n377 = call <vilib>:"WPI_MotorControlRefNum Registry Get.vi"("refnum name"="polea") -> ("error out"=w676:errorcluster, "MotorControlDevRef"=w675:T6)  [unwired: 9 in]
                n378 = Wait (ms)(milliseconds to wait=u32 200) -> ()  [unwired: 1 out]
                n379 = call <vilib>:"WPI_MotorControlSetOutput.vi"("error in (no error)"=w676, "Output"=-0.5 ("Motor Output"), "MotorControlDevRef"=w675) -> ()  [unwired: 6 in, 3 out]
              }
              frame #1 {
                n380 = call <vilib>:"WPI_MotorControlRefNum Registry Get.vi"("refnum name"="polea") -> ("error out"=w680:errorcluster, "MotorControlDevRef"=w679:T6)  [unwired: 9 in]
                n381 = call <vilib>:"WPI_MotorControlRefNum Registry Get.vi"("refnum name"="bomberos") -> ("error out"=w684:errorcluster, "MotorControlDevRef"=w683:T6)  [unwired: 9 in]
                n382 = call <vilib>:"WPI_MotorControlSetOutput.vi"("error in (no error)"=w680, "Output"=0.0 ("Motor Output"), "MotorControlDevRef"=w679) -> ()  [unwired: 6 in, 3 out]
                n383 = call <vilib>:"WPI_MotorControlSetOutput.vi"("error in (no error)"=w684, "Output"=0.5 ("Motor Output"), "MotorControlDevRef"=w683) -> ()  [unwired: 6 in, 3 out]
              }
              frame #2 {
                n384 = call <vilib>:"WPI_MotorControlRefNum Registry Get.vi"("refnum name"="bomberos") -> ("error out"=w687:errorcluster, "MotorControlDevRef"=w688:T6)  [unwired: 9 in]
                n385 = call <vilib>:"WPI_MotorControlSetOutput.vi"("error in (no error)"=w687, "Output"=0.0 ("Motor Output"), "MotorControlDevRef"=w688) -> ()  [unwired: 6 in, 3 out]
              }
              frame #3 {
              }
            }
          }
          frame 2 {
            n386 = flat-sequence {
              tunnel: [3.0] -> w690
              frame #0 {
                n387 = call <vilib>:"WPI_SolenoidRefNum Registry Get.vi"("refnum name"="pickup") -> ("SolenoidDevRef"=w693:T11)  [unwired: 9 in, 1 out]
                n388 = call-poly <vilib>:"WPI_SolenoidSet.vi"("Value"=WPI_SolenoidValue."Forward", "SolenoidDevRef"=w693) -> ()  [unwired: 8 in, 2 out]
                n389 = Wait (ms)(milliseconds to wait=u32 200) -> ()  [unwired: 1 out]
              }
              frame #1 {
              }
            }
          }
          frame 3 {
            n390 = flat-sequence {
              tunnel: [4.0] -> w696
              frame #0 {
                n391 = call <vilib>:"WPI_RobotDriveRefNum Registry Get.vi"("refnum name"="chasis") -> ("error out"=w700:errorcluster, "RobotDriveDevRef"=w701:T13)  [unwired: 9 in]
                n392 = call-poly <vilib>:"WPI_RobotDriveArcadeDrive.vi"("error in (no error)"=w700, "Y axis value"=-0.5 ("Motor Output"), "X axis value"=0.5 ("Motor Output"), "RobotDriveDevRef"=w701) -> ("error out"=w699:errorcluster, "RobotDriveDevRef"=w698:T13)  [unwired: 5 in, 1 out]
                n393 = call <vilib>:"WPI_RobotDriveDelayAndUpdateSafety.vi"("error in (no error)"=w699, "Delay (s)"=3.0, "RobotDriveDevRef"=w698) -> ()  [unwired: 7 in, 2 out]
              }
              frame #1 {
                n394 = call <vilib>:"WPI_RobotDriveRefNum Registry Get.vi"("refnum name"="chasis") -> ("error out"=w708:errorcluster, "RobotDriveDevRef"=w709:T13)  [unwired: 9 in]
                n395 = call-poly <vilib>:"WPI_RobotDriveArcadeDrive.vi"("error in (no error)"=w708, "Y axis value"=0.5 ("Motor Output"), "X axis value"=0.5 ("Motor Output"), "RobotDriveDevRef"=w709) -> ("error out"=w706:errorcluster, "RobotDriveDevRef"=w707:T13)  [unwired: 5 in, 1 out]
                n396 = call <vilib>:"WPI_RobotDriveDelayAndUpdateSafety.vi"("error in (no error)"=w706, "Delay (s)"=2.0, "RobotDriveDevRef"=w707) -> ()  [unwired: 7 in, 2 out]
              }
              frame #2 {
                w715 = 0.0 ("Motor Output")
                n397 = call <vilib>:"WPI_RobotDriveRefNum Registry Get.vi"("refnum name"="chasis") -> ("error out"=w713:errorcluster, "RobotDriveDevRef"=w714:T13)  [unwired: 9 in]
                n398 = call-poly <vilib>:"WPI_RobotDriveArcadeDrive.vi"("error in (no error)"=w713, "Y axis value"=w715, "X axis value"=w715, "RobotDriveDevRef"=w714) -> ()  [unwired: 5 in, 3 out]
              }
              frame #3 {
              }
            }
          }
          frame 4 {
            n399 = flat-sequence {
              tunnel: [5.0] -> w718
              frame #0 {
                n400 = call <vilib>:"WPI_MotorControlRefNum Registry Get.vi"("refnum name"="bomberos") -> ("error out"=w727:errorcluster, "MotorControlDevRef"=w726:T6)  [unwired: 9 in]
                n401 = call <vilib>:"WPI_MotorControlSetOutput.vi"("error in (no error)"=w727, "Output"=-0.5 ("Motor Output"), "MotorControlDevRef"=w726) -> ()  [unwired: 6 in, 3 out]
                n402 = Wait (ms)(milliseconds to wait=u32 20) -> ()  [unwired: 1 out]
                n403 = call <vilib>:"WPI_MotorControlRefNum Registry Get.vi"("refnum name"="polea") -> ("error out"=w723:errorcluster, "MotorControlDevRef"=w722:T6)  [unwired: 9 in]
                n404 = call <vilib>:"WPI_MotorControlSetOutput.vi"("error in (no error)"=w723, "Output"=0.5 ("Motor Output"), "MotorControlDevRef"=w722) -> ()  [unwired: 6 in, 3 out]
              }
              frame #1 {
                n405 = call <vilib>:"WPI_MotorControlRefNum Registry Get.vi"("refnum name"="polea") -> ("error out"=w734:errorcluster, "MotorControlDevRef"=w735:T6)  [unwired: 9 in]
                n406 = call <vilib>:"WPI_MotorControlRefNum Registry Get.vi"("refnum name"="bomberos") -> ("error out"=w732:errorcluster, "MotorControlDevRef"=w733:T6)  [unwired: 9 in]
                n407 = call <vilib>:"WPI_MotorControlSetOutput.vi"("error in (no error)"=w734, "Output"=0.0 ("Motor Output"), "MotorControlDevRef"=w735) -> ()  [unwired: 6 in, 3 out]
                n408 = call <vilib>:"WPI_MotorControlSetOutput.vi"("error in (no error)"=w732, "Output"=0.0 ("Motor Output"), "MotorControlDevRef"=w733) -> ()  [unwired: 6 in, 3 out]
              }
              frame #2 {
              }
            }
          }
          frame 5 {
            n409 = flat-sequence {
              tunnel: [6.0] -> w737
              frame #0 {
                n410 = call <vilib>:"WPI_SolenoidRefNum Registry Get.vi"("refnum name"="pickup") -> ("SolenoidDevRef"=w740:T11)  [unwired: 9 in, 1 out]
                n411 = call-poly <vilib>:"WPI_SolenoidSet.vi"("Value"=WPI_SolenoidValue."Forward", "SolenoidDevRef"=w740) -> ()  [unwired: 8 in, 2 out]
                n412 = Wait (ms)(milliseconds to wait=u32 200) -> ()  [unwired: 1 out]
              }
              frame #1 {
              }
            }
          }
          frame 6 {
            n413 = flat-sequence {
              tunnel: [7.0] -> w743
              frame #0 {
                n414 = call <vilib>:"WPI_MotorControlRefNum Registry Get.vi"("refnum name"="polea") -> ("error out"=w752:errorcluster, "MotorControlDevRef"=w751:T6)  [unwired: 9 in]
                n415 = Wait (ms)(milliseconds to wait=u32 30) -> ()  [unwired: 1 out]
                n416 = call <vilib>:"WPI_MotorControlSetOutput.vi"("error in (no error)"=w752, "Output"=-0.5, "MotorControlDevRef"=w751) -> ()  [unwired: 6 in, 3 out]
                n417 = call <vilib>:"WPI_MotorControlRefNum Registry Get.vi"("refnum name"="bomberos") -> ("error out"=w748:errorcluster, "MotorControlDevRef"=w747:T6)  [unwired: 9 in]
                n418 = call <vilib>:"WPI_MotorControlSetOutput.vi"("error in (no error)"=w748, "Output"=-0.5, "MotorControlDevRef"=w747) -> ()  [unwired: 6 in, 3 out]
              }
              frame #1 {
                n419 = call <vilib>:"WPI_MotorControlRefNum Registry Get.vi"("refnum name"="polea") -> ("error out"=w759:errorcluster, "MotorControlDevRef"=w760:T6)  [unwired: 9 in]
                n420 = call <vilib>:"WPI_MotorControlRefNum Registry Get.vi"("refnum name"="bomberos") -> ("error out"=w755:errorcluster, "MotorControlDevRef"=w756:T6)  [unwired: 9 in]
                n421 = call <vilib>:"WPI_MotorControlSetOutput.vi"("error in (no error)"=w759, "Output"=0.0, "MotorControlDevRef"=w760) -> ()  [unwired: 6 in, 3 out]
                n422 = call <vilib>:"WPI_MotorControlSetOutput.vi"("error in (no error)"=w755, "Output"=0.0, "MotorControlDevRef"=w756) -> ()  [unwired: 6 in, 3 out]
              }
              frame #2 {
              }
            }
          }
          frame 7 {
            n423 = flat-sequence {
              tunnel: [8.0] -> w762
              frame #0 {
                n424 = call <vilib>:"WPI_RobotDriveRefNum Registry Get.vi"("refnum name"="chasis") -> ("error out"=w766:errorcluster, "RobotDriveDevRef"=w767:T13)  [unwired: 9 in]
                n425 = call-poly <vilib>:"WPI_RobotDriveArcadeDrive.vi"("error in (no error)"=w766, "Y axis value"=-0.5 ("Motor Output"), "X axis value"=0.5 ("Motor Output"), "RobotDriveDevRef"=w767) -> ("error out"=w764:errorcluster, "RobotDriveDevRef"=w765:T13)  [unwired: 5 in, 1 out]
                n426 = call <vilib>:"WPI_RobotDriveDelayAndUpdateSafety.vi"("error in (no error)"=w764, "Delay (s)"=29.0, "RobotDriveDevRef"=w765) -> ()  [unwired: 7 in, 2 out]
              }
              frame #1 {
                n427 = call <vilib>:"WPI_RobotDriveRefNum Registry Get.vi"("refnum name"="chasis") -> ("error out"=w775:errorcluster, "RobotDriveDevRef"=w776:T13)  [unwired: 9 in]
                n428 = call-poly <vilib>:"WPI_RobotDriveArcadeDrive.vi"("error in (no error)"=w775, "Y axis value"=0.5 ("Motor Output"), "X axis value"=0.5 ("Motor Output"), "RobotDriveDevRef"=w776) -> ("error out"=w773:errorcluster, "RobotDriveDevRef"=w772:T13)  [unwired: 5 in, 1 out]
                n429 = call <vilib>:"WPI_RobotDriveDelayAndUpdateSafety.vi"("error in (no error)"=w773, "Delay (s)"=29.0, "RobotDriveDevRef"=w772) -> ()  [unwired: 7 in, 2 out]
              }
              frame #2 {
                w779 = 0.0 ("Motor Output")
                n430 = call <vilib>:"WPI_RobotDriveRefNum Registry Get.vi"("refnum name"="chasis") -> ("error out"=w780:errorcluster, "RobotDriveDevRef"=w781:T13)  [unwired: 9 in]
                n431 = call-poly <vilib>:"WPI_RobotDriveArcadeDrive.vi"("error in (no error)"=w780, "Y axis value"=w779, "X axis value"=w779, "RobotDriveDevRef"=w781) -> ()  [unwired: 5 in, 3 out]
              }
              frame #3 {
              }
            }
          }
          frame 8 {
            n432 = flat-sequence {
              tunnel: [9.0] -> w784
              frame #0 {
                n433 = call <vilib>:"WPI_MotorControlRefNum Registry Get.vi"("refnum name"="polea") -> ("error out"=w793:errorcluster, "MotorControlDevRef"=w792:T6)  [unwired: 9 in]
                n434 = Wait (ms)(milliseconds to wait=u32 30) -> ()  [unwired: 1 out]
                n435 = call <vilib>:"WPI_MotorControlSetOutput.vi"("error in (no error)"=w793, "Output"=0.5, "MotorControlDevRef"=w792) -> ()  [unwired: 6 in, 3 out]
                n436 = call <vilib>:"WPI_MotorControlRefNum Registry Get.vi"("refnum name"="bomberos") -> ("error out"=w789:errorcluster, "MotorControlDevRef"=w788:T6)  [unwired: 9 in]
                n437 = call <vilib>:"WPI_MotorControlSetOutput.vi"("error in (no error)"=w789, "Output"=-0.5, "MotorControlDevRef"=w788) -> ()  [unwired: 6 in, 3 out]
              }
              frame #1 {
                n438 = call <vilib>:"WPI_MotorControlRefNum Registry Get.vi"("refnum name"="polea") -> ("error out"=w800:errorcluster, "MotorControlDevRef"=w801:T6)  [unwired: 9 in]
                n439 = call <vilib>:"WPI_MotorControlRefNum Registry Get.vi"("refnum name"="bomberos") -> ("error out"=w796:errorcluster, "MotorControlDevRef"=w797:T6)  [unwired: 9 in]
                n440 = call <vilib>:"WPI_MotorControlSetOutput.vi"("error in (no error)"=w800, "Output"=0.0, "MotorControlDevRef"=w801) -> ()  [unwired: 6 in, 3 out]
                n441 = call <vilib>:"WPI_MotorControlSetOutput.vi"("error in (no error)"=w796, "Output"=0.0, "MotorControlDevRef"=w797) -> ()  [unwired: 6 in, 3 out]
              }
              frame #2 {
              }
            }
          }
          frame 9 {
            n442 = flat-sequence {
              tunnel: [9.0] -> w804
              tunnel: [FALSE] -> w803
              frame #0 {
                n443 = call <vilib>:"WPI_SolenoidRefNum Registry Get.vi"("refnum name"="pickup") -> ("SolenoidDevRef"=w807:T11)  [unwired: 9 in, 1 out]
                n444 = call-poly <vilib>:"WPI_SolenoidSet.vi"("Value"=WPI_SolenoidValue."Reverse", "SolenoidDevRef"=w807) -> ()  [unwired: 8 in, 2 out]
                n445 = Wait (ms)(milliseconds to wait=u32 200) -> ()  [unwired: 1 out]
              }
              frame #1 {
              }
            }
          }
        }
      }
    }
    frame "Caso2-pos1" {
      n446 = while {
        shift-right: [w813] -> _
        shift-left: 1.0 -> [w814]
        stop <- w812 stop-if-true
        n447 = case shown="8" w814 {
          tunnel: [1.0 w816 w849 w855 w885 w918 w924 w957 w987 w1021] -> w813
          tunnel: [_ _ _ _ _ _ _ _ _ w1020] -> w812
          frame 0, Default {
          }
          frame 1 {
            n448 = flat-sequence {
              tunnel: [2.0] -> w816
              frame #0 {
                n449 = call <vilib>:"WPI_MotorControlRefNum Registry Get.vi"("refnum name"="bomberos") -> ("error out"=w817:errorcluster, "MotorControlDevRef"=w818:T6)  [unwired: 9 in]
                n450 = call <vilib>:"WPI_MotorControlRefNum Registry Get.vi"("refnum name"="polea") -> ("error out"=w821:errorcluster, "MotorControlDevRef"=w822:T6)  [unwired: 9 in]
                n451 = call <vilib>:"Spark MAX Set Sensor Position.vi"("error in"=w817, "Position"=0.0, "MotorControlDeviceRef"=w818) -> ()  [unwired: 7 in, 2 out]
                n452 = call <vilib>:"Spark MAX Set Sensor Position.vi"("error in"=w821, "Position"=0.0, "MotorControlDeviceRef"=w822) -> ()  [unwired: 7 in, 2 out]
              }
              frame #1 {
                n453 = while {
                  stop <- w828 stop-if-true
                  n454 = call <vilib>:"WPI_MotorControlRefNum Registry Get.vi"("refnum name"="polea") -> ("error out"=w838:errorcluster, "MotorControlDevRef"=w839:T6)  [unwired: 9 in]
                  n455 = global read "Robot Global Data.vi" "bomberos"() -> (w827:dbl)
                  n456 = global read "Robot Global Data.vi" "vpolea"() -> (w835:dbl)
                  n457 = call <vilib>:"WPI_MotorControlSetOutput.vi"("error in (no error)"=w838, "Output"=-0.5 ("Motor Output"), "MotorControlDevRef"=w839) -> ()  [unwired: 6 in, 3 out]
                  n458 = Greater Or Equal?(x=w827, y=15.0) -> (x >= y?=w825:bool)
                  n459 = Greater Or Equal?(x=w835, y=15.0) -> (x >= y?=w829:bool)
                  n460 = call <vilib>:"WPI_MotorControlRefNum Registry Get.vi"("refnum name"="bomberos") -> ("error out"=w833:errorcluster, "MotorControlDevRef"=w832:T6)  [unwired: 9 in]
                  n461 = And(x=w829, y=w825) -> (x .and. y?=w828:bool)
                  n462 = call <vilib>:"WPI_MotorControlSetOutput.vi"("error in (no error)"=w833, "Output"=0.5 ("Motor Output"), "MotorControlDevRef"=w832) -> ()  [unwired: 6 in, 3 out]
                }
              }
              frame #2 {
                n463 = call <vilib>:"WPI_MotorControlRefNum Registry Get.vi"("refnum name"="bomberos") -> ("error out"=w842:errorcluster, "MotorControlDevRef"=w843:T6)  [unwired: 9 in]
                n464 = call <vilib>:"WPI_MotorControlRefNum Registry Get.vi"("refnum name"="polea") -> ("error out"=w846:errorcluster, "MotorControlDevRef"=w847:T6)  [unwired: 9 in]
                n465 = call <vilib>:"WPI_MotorControlSetOutput.vi"("error in (no error)"=w842, "Output"=0.0 ("Motor Output"), "MotorControlDevRef"=w843) -> ()  [unwired: 6 in, 3 out]
                n466 = call <vilib>:"WPI_MotorControlSetOutput.vi"("error in (no error)"=w846, "Output"=0.0 ("Motor Output"), "MotorControlDevRef"=w847) -> ()  [unwired: 6 in, 3 out]
              }
              frame #3 {
              }
            }
          }
          frame 2 {
            n467 = flat-sequence {
              tunnel: [3.0] -> w849
              frame #0 {
                n468 = call <vilib>:"WPI_SolenoidRefNum Registry Get.vi"("refnum name"="pickup") -> ("SolenoidDevRef"=w852:T11)  [unwired: 9 in, 1 out]
                n469 = call-poly <vilib>:"WPI_SolenoidSet.vi"("Value"=WPI_SolenoidValue."Reverse", "SolenoidDevRef"=w852) -> ()  [unwired: 8 in, 2 out]
                n470 = Wait (ms)(milliseconds to wait=u32 200) -> ()  [unwired: 1 out]
              }
              frame #1 {
              }
            }
          }
          frame 3 {
            n471 = flat-sequence {
              tunnel: [4.0] -> w855
              frame #0 {
                n472 = call <vilib>:"WPI_MotorControlRefNum Registry Get.vi"("refnum name"="llantas") -> ("error out"=w856:errorcluster, "MotorControlDevRef"=w857:T6)  [unwired: 9 in]
                n473 = call <vilib>:"Spark MAX Set Sensor Position.vi"("error in"=w856, "Position"=0.0, "MotorControlDeviceRef"=w857) -> ()  [unwired: 7 in, 2 out]
              }
              frame #1 {
                n474 = while {
                  stop <- w864 stop-if-true
                  # "da vuelta"
                  n475 = global read "Robot Global Data.vi" "ruedaiz"() -> (w866:dbl)
                  n476 = call <vilib>:"WPI_RobotDriveRefNum Registry Get.vi"("refnum name"="chasis") -> ("error out"=w860:errorcluster, "RobotDriveDevRef"=w861:T13)  [unwired: 9 in]
                  n477 = Greater Or Equal?(x=w866, y=40.0) -> (x >= y?=w864:bool)
                  n478 = call-poly <vilib>:"WPI_RobotDriveArcadeDrive.vi"("error in (no error)"=w860, "Y axis value"=-0.5 ("Motor Output"), "X axis value"=0.5 ("Motor Output"), "RobotDriveDevRef"=w861) -> ()  [unwired: 5 in, 3 out]
                }
              }
              frame #2 {
                n479 = call <vilib>:"WPI_MotorControlRefNum Registry Get.vi"("refnum name"="llantas") -> ("error out"=w868:errorcluster, "MotorControlDevRef"=w869:T6)  [unwired: 9 in]
                n480 = call <vilib>:"Spark MAX Set Sensor Position.vi"("error in"=w868, "Position"=0.0, "MotorControlDeviceRef"=w869) -> ()  [unwired: 7 in, 2 out]
              }
              frame #3 {
                n481 = while {
                  stop <- w876 stop-if-true
                  # "avanza"
                  n482 = global read "Robot Global Data.vi" "ruedaiz"() -> (w878:dbl)
                  n483 = call <vilib>:"WPI_RobotDriveRefNum Registry Get.vi"("refnum name"="chasis") -> ("error out"=w872:errorcluster, "RobotDriveDevRef"=w873:T13)  [unwired: 9 in]
                  n484 = Greater Or Equal?(x=w878, y=50.0) -> (x >= y?=w876:bool)
                  n485 = call-poly <vilib>:"WPI_RobotDriveArcadeDrive.vi"("error in (no error)"=w872, "Y axis value"=0.5 ("Motor Output"), "X axis value"=0.5 ("Motor Output"), "RobotDriveDevRef"=w873) -> ()  [unwired: 5 in, 3 out]
                }
              }
              frame #4 {
                w882 = 0.0 ("Motor Output")
                n486 = call <vilib>:"WPI_RobotDriveRefNum Registry Get.vi"("refnum name"="chasis") -> ("error out"=w880:errorcluster, "RobotDriveDevRef"=w881:T13)  [unwired: 9 in]
                n487 = call-poly <vilib>:"WPI_RobotDriveArcadeDrive.vi"("error in (no error)"=w880, "Y axis value"=w882, "X axis value"=w882, "RobotDriveDevRef"=w881) -> ()  [unwired: 5 in, 3 out]
              }
              frame #5 {
              }
            }
          }
          frame 4 {
            n488 = flat-sequence {
              tunnel: [5.0] -> w885
              frame #0 {
                n489 = call <vilib>:"WPI_MotorControlRefNum Registry Get.vi"("refnum name"="polea") -> ("error out"=w886:errorcluster, "MotorControlDevRef"=w887:T6)  [unwired: 9 in]
                n490 = call <vilib>:"Spark MAX Set Sensor Position.vi"("error in"=w886, "Position"=0.0, "MotorControlDeviceRef"=w887) -> ()  [unwired: 7 in, 2 out]
                n491 = call <vilib>:"WPI_MotorControlRefNum Registry Get.vi"("refnum name"="bomberos") -> ("error out"=w890:errorcluster, "MotorControlDevRef"=w891:T6)  [unwired: 9 in]
                n492 = call <vilib>:"Spark MAX Set Sensor Position.vi"("error in"=w890, "Position"=0.0, "MotorControlDeviceRef"=w891) -> ()  [unwired: 7 in, 2 out]
              }
              frame #1 {
                n493 = while {
                  stop <- w898 stop-if-true
                  n494 = global read "Robot Global Data.vi" "bomberos"() -> (w900:dbl)
                  n495 = call <vilib>:"WPI_MotorControlRefNum Registry Get.vi"("refnum name"="bomberos") -> ("error out"=w908:errorcluster, "MotorControlDevRef"=w907:T6)  [unwired: 9 in]
                  n496 = global read "Robot Global Data.vi" "vpolea"() -> (w896:dbl)
                  n497 = call <vilib>:"WPI_MotorControlSetOutput.vi"("error in (no error)"=w908, "Output"=-0.5 ("Motor Output"), "MotorControlDevRef"=w907) -> ()  [unwired: 6 in, 3 out]
                  n498 = Greater Or Equal?(x=w900, y=20.0) -> (x >= y?=w899:bool)
                  n499 = Greater Or Equal?(x=w896, y=20.0) -> (x >= y?=w894:bool)
                  n500 = call <vilib>:"WPI_MotorControlRefNum Registry Get.vi"("refnum name"="polea") -> ("error out"=w904:errorcluster, "MotorControlDevRef"=w903:T6)  [unwired: 9 in]
                  n501 = And(x=w899, y=w894) -> (x .and. y?=w898:bool)
                  n502 = call <vilib>:"WPI_MotorControlSetOutput.vi"("error in (no error)"=w904, "Output"=0.5 ("Motor Output"), "MotorControlDevRef"=w903) -> ()  [unwired: 6 in, 3 out]
                }
              }
              frame #2 {
                n503 = call <vilib>:"WPI_MotorControlRefNum Registry Get.vi"("refnum name"="polea") -> ("error out"=w915:errorcluster, "MotorControlDevRef"=w916:T6)  [unwired: 9 in]
                n504 = call <vilib>:"WPI_MotorControlRefNum Registry Get.vi"("refnum name"="bomberos") -> ("error out"=w913:errorcluster, "MotorControlDevRef"=w914:T6)  [unwired: 9 in]
                n505 = call <vilib>:"WPI_MotorControlSetOutput.vi"("error in (no error)"=w915, "Output"=0.0 ("Motor Output"), "MotorControlDevRef"=w916) -> ()  [unwired: 6 in, 3 out]
                n506 = call <vilib>:"WPI_MotorControlSetOutput.vi"("error in (no error)"=w913, "Output"=0.0 ("Motor Output"), "MotorControlDevRef"=w914) -> ()  [unwired: 6 in, 3 out]
              }
              frame #3 {
              }
            }
          }
          frame 5 {
            n507 = flat-sequence {
              tunnel: [6.0] -> w918
              frame #0 {
                n508 = Wait (ms)(milliseconds to wait=u32 200) -> ()  [unwired: 1 out]
                n509 = call <vilib>:"WPI_SolenoidRefNum Registry Get.vi"("refnum name"="pickup") -> ("SolenoidDevRef"=w922:T11)  [unwired: 9 in, 1 out]
                n510 = call-poly <vilib>:"WPI_SolenoidSet.vi"("Value"=WPI_SolenoidValue."Forward", "SolenoidDevRef"=w922) -> ()  [unwired: 8 in, 2 out]
              }
              frame #1 {
              }
            }
          }
          frame 6 {
            n511 = flat-sequence {
              tunnel: [7.0] -> w924
              frame #0 {
                n512 = call <vilib>:"WPI_MotorControlRefNum Registry Get.vi"("refnum name"="bomberos") -> ("error out"=w929:errorcluster, "MotorControlDevRef"=w930:T6)  [unwired: 9 in]
                n513 = call <vilib>:"WPI_MotorControlRefNum Registry Get.vi"("refnum name"="polea") -> ("error out"=w925:errorcluster, "MotorControlDevRef"=w926:T6)  [unwired: 9 in]
                n514 = call <vilib>:"Spark MAX Set Sensor Position.vi"("error in"=w929, "Position"=0.0, "MotorControlDeviceRef"=w930) -> ()  [unwired: 7 in, 2 out]
                n515 = call <vilib>:"Spark MAX Set Sensor Position.vi"("error in"=w925, "Position"=0.0, "MotorControlDeviceRef"=w926) -> ()  [unwired: 7 in, 2 out]
              }
              frame #1 {
                n516 = while {
                  stop <- w936 stop-if-true
                  n517 = global read "Robot Global Data.vi" "bomberos"() -> (w935:dbl)
                  n518 = global read "Robot Global Data.vi" "vpolea"() -> (w943:dbl)
                  n519 = call <vilib>:"WPI_MotorControlRefNum Registry Get.vi"("refnum name"="polea") -> ("error out"=w947:errorcluster, "MotorControlDevRef"=w946:T6)  [unwired: 9 in]
                  n520 = Equal?(x=w935, y=15.0) -> (x = y?=w933:bool)
                  n521 = call <vilib>:"WPI_MotorControlSetOutput.vi"("error in (no error)"=w947, "Output"=-0.5, "MotorControlDevRef"=w946) -> ()  [unwired: 6 in, 3 out]
                  n522 = Equal?(x=w943, y=15.0) -> (x = y?=w937:bool)
                  n523 = call <vilib>:"WPI_MotorControlRefNum Registry Get.vi"("refnum name"="bomberos") -> ("error out"=w941:errorcluster, "MotorControlDevRef"=w940:T6)  [unwired: 9 in]
                  n524 = And(x=w937, y=w933) -> (x .and. y?=w936:bool)
                  n525 = call <vilib>:"WPI_MotorControlSetOutput.vi"("error in (no error)"=w941, "Output"=-0.5, "MotorControlDevRef"=w940) -> ()  [unwired: 6 in, 3 out]
                }
              }
              frame #2 {
                n526 = call <vilib>:"WPI_MotorControlRefNum Registry Get.vi"("refnum name"="polea") -> ("error out"=w954:errorcluster, "MotorControlDevRef"=w955:T6)  [unwired: 9 in]
                n527 = call <vilib>:"WPI_MotorControlRefNum Registry Get.vi"("refnum name"="bomberos") -> ("error out"=w950:errorcluster, "MotorControlDevRef"=w951:T6)  [unwired: 9 in]
                n528 = call <vilib>:"WPI_MotorControlSetOutput.vi"("error in (no error)"=w954, "Output"=0.0, "MotorControlDevRef"=w955) -> ()  [unwired: 6 in, 3 out]
                n529 = call <vilib>:"WPI_MotorControlSetOutput.vi"("error in (no error)"=w950, "Output"=0.0, "MotorControlDevRef"=w951) -> ()  [unwired: 6 in, 3 out]
              }
              frame #3 {
              }
            }
          }
          frame 7 {
            n530 = flat-sequence {
              tunnel: [8.0] -> w957
              frame #0 {
                n531 = call <vilib>:"WPI_MotorControlRefNum Registry Get.vi"("refnum name"="llanta") -> ("error out"=w958:errorcluster, "MotorControlDevRef"=w959:T6)  [unwired: 9 in]
                n532 = call <vilib>:"Spark MAX Set Sensor Position.vi"("error in"=w958, "Position"=0.0, "MotorControlDeviceRef"=w959) -> ()  [unwired: 7 in, 2 out]
              }
              frame #1 {
                n533 = while {
                  stop <- w966 stop-if-true
                  # "da vuelta"
                  n534 = global read "Robot Global Data.vi" "ruedaiz"() -> (w968:dbl)
                  n535 = call <vilib>:"WPI_RobotDriveRefNum Registry Get.vi"("refnum name"="chasis") -> ("error out"=w962:errorcluster, "RobotDriveDevRef"=w963:T13)  [unwired: 9 in]
                  n536 = Equal?(x=w968, y=40.0) -> (x = y?=w966:bool)
                  n537 = call-poly <vilib>:"WPI_RobotDriveArcadeDrive.vi"("error in (no error)"=w962, "Y axis value"=-0.5 ("Motor Output"), "X axis value"=0.5 ("Motor Output"), "RobotDriveDevRef"=w963) -> ()  [unwired: 5 in, 3 out]
                }
              }
              frame #2 {
                n538 = call <vilib>:"WPI_MotorControlRefNum Registry Get.vi"("refnum name"="llanta") -> ("error out"=w970:errorcluster, "MotorControlDevRef"=w971:T6)  [unwired: 9 in]
                n539 = call <vilib>:"Spark MAX Set Sensor Position.vi"("error in"=w970, "Position"=0.0, "MotorControlDeviceRef"=w971) -> ()  [unwired: 7 in, 2 out]
              }
              frame #3 {
                n540 = while {
                  stop <- w978 stop-if-true
                  # "avanza"
                  n541 = global read "Robot Global Data.vi" "ruedaiz"() -> (w980:dbl)
                  n542 = call <vilib>:"WPI_RobotDriveRefNum Registry Get.vi"("refnum name"="chasis") -> ("error out"=w974:errorcluster, "RobotDriveDevRef"=w975:T13)  [unwired: 9 in]
                  n543 = Equal?(x=w980, y=50.0) -> (x = y?=w978:bool)
                  n544 = call-poly <vilib>:"WPI_RobotDriveArcadeDrive.vi"("error in (no error)"=w974, "Y axis value"=0.5 ("Motor Output"), "X axis value"=0.5 ("Motor Output"), "RobotDriveDevRef"=w975) -> ()  [unwired: 5 in, 3 out]
                }
              }
              frame #4 {
                w982 = 0.0 ("Motor Output")
                n545 = call <vilib>:"WPI_RobotDriveRefNum Registry Get.vi"("refnum name"="chasis") -> ("error out"=w983:errorcluster, "RobotDriveDevRef"=w984:T13)  [unwired: 9 in]
                n546 = call-poly <vilib>:"WPI_RobotDriveArcadeDrive.vi"("error in (no error)"=w983, "Y axis value"=w982, "X axis value"=w982, "RobotDriveDevRef"=w984) -> ()  [unwired: 5 in, 3 out]
              }
              frame #5 {
              }
            }
          }
          frame 8 {
            n547 = flat-sequence {
              tunnel: [9.0] -> w987
              frame #0 {
                n548 = call <vilib>:"WPI_MotorControlRefNum Registry Get.vi"("refnum name"="bomberos") -> ("error out"=w992:errorcluster, "MotorControlDevRef"=w993:T6)  [unwired: 9 in]
                n549 = call <vilib>:"WPI_MotorControlRefNum Registry Get.vi"("refnum name"="polea") -> ("error out"=w988:errorcluster, "MotorControlDevRef"=w989:T6)  [unwired: 9 in]
                n550 = call <vilib>:"Spark MAX Set Sensor Position.vi"("error in"=w992, "Position"=0.0, "MotorControlDeviceRef"=w993) -> ()  [unwired: 7 in, 2 out]
                n551 = call <vilib>:"Spark MAX Set Sensor Position.vi"("error in"=w988, "Position"=0.0, "MotorControlDeviceRef"=w989) -> ()  [unwired: 7 in, 2 out]
              }
              frame #1 {
                n552 = while {
                  stop <- w999 stop-if-true
                  n553 = global read "Robot Global Data.vi" "bomberos"() -> (w998:dbl)
                  n554 = global read "Robot Global Data.vi" "vpolea"() -> (w1006:dbl)
                  n555 = call <vilib>:"WPI_MotorControlRefNum Registry Get.vi"("refnum name"="polea") -> ("error out"=w1010:errorcluster, "MotorControlDevRef"=w1009:T6)  [unwired: 9 in]
                  n556 = Equal?(x=w998, y=15.0) -> (x = y?=w996:bool)
                  n557 = call <vilib>:"WPI_MotorControlSetOutput.vi"("error in (no error)"=w1010, "Output"=-0.5, "MotorControlDevRef"=w1009) -> ()  [unwired: 6 in, 3 out]
                  n558 = Equal?(x=w1006, y=15.0) -> (x = y?=w1000:bool)
                  n559 = call <vilib>:"WPI_MotorControlRefNum Registry Get.vi"("refnum name"="bomberos") -> ("error out"=w1004:errorcluster, "MotorControlDevRef"=w1003:T6)  [unwired: 9 in]
                  n560 = And(x=w1000, y=w996) -> (x .and. y?=w999:bool)
                  n561 = call <vilib>:"WPI_MotorControlSetOutput.vi"("error in (no error)"=w1004, "Output"=-0.5, "MotorControlDevRef"=w1003) -> ()  [unwired: 6 in, 3 out]
                }
              }
              frame #2 {
                n562 = call <vilib>:"WPI_MotorControlRefNum Registry Get.vi"("refnum name"="polea") -> ("error out"=w1017:errorcluster, "MotorControlDevRef"=w1018:T6)  [unwired: 9 in]
                n563 = call <vilib>:"WPI_MotorControlRefNum Registry Get.vi"("refnum name"="bomberos") -> ("error out"=w1013:errorcluster, "MotorControlDevRef"=w1014:T6)  [unwired: 9 in]
                n564 = call <vilib>:"WPI_MotorControlSetOutput.vi"("error in (no error)"=w1017, "Output"=0.0, "MotorControlDevRef"=w1018) -> ()  [unwired: 6 in, 3 out]
                n565 = call <vilib>:"WPI_MotorControlSetOutput.vi"("error in (no error)"=w1013, "Output"=0.0, "MotorControlDevRef"=w1014) -> ()  [unwired: 6 in, 3 out]
              }
              frame #3 {
              }
            }
          }
          frame 9 {
            n566 = flat-sequence {
              tunnel: [10.0] -> w1021
              tunnel: [FALSE] -> w1020
              frame #0 {
                n567 = call <vilib>:"WPI_SolenoidRefNum Registry Get.vi"("refnum name"="pickup") -> ("SolenoidDevRef"=w1024:T11)  [unwired: 9 in, 1 out]
                n568 = call-poly <vilib>:"WPI_SolenoidSet.vi"("Value"=WPI_SolenoidValue."Reverse", "SolenoidDevRef"=w1024) -> ()  [unwired: 8 in, 2 out]
                n569 = Wait (ms)(milliseconds to wait=u32 200) -> ()  [unwired: 1 out]
              }
              frame #1 {
              }
            }
          }
        }
      }
    }
    frame "supreme" {
      n570 = while {
        shift-right: [w1030] -> _
        shift-left: 1.0 -> [w1031]
        stop <- w1029 stop-if-true
        n571 = case shown="2" w1031 {
          tunnel: [1.0 w1033 w1054] -> w1030
          tunnel: [_ _ w1053] -> w1029
          frame 0, Default {
          }
          frame 1 {
            n572 = flat-sequence {
              tunnel: [2.0] -> w1033
              frame #0 {
                n573 = while {
                  stop <- w1037 stop-if-true
                  w1034 = -0.2 ("Motor Output")
                  n574 = global read "Robot Global Data.vi" "ruedaiz"() -> (w1039:dbl)
                  n575 = call <vilib>:"WPI_RobotDriveRefNum Registry Get.vi"("refnum name"="chasis") -> ("error out"=w1035:errorcluster, "RobotDriveDevRef"=w1036:T13)  [unwired: 9 in]
                  n576 = Greater Or Equal?(x=w1039, y=10.0) -> (x >= y?=w1037:bool)
                  n577 = call <vilib>:"WPI_RobotDriveTankDrive.vi"("error in (no error)"=w1035, "Right axis value"=w1034, "Left axis value"=w1034, "RobotDriveDevRef"=w1036) -> ()  [unwired: 5 in, 3 out]
                }
              }
              frame #1 {
                n578 = while {
                  stop <- w1044 stop-if-true
                  w1041 = 0.8 ("Motor Output")
                  n579 = global read "Robot Global Data.vi" "ruedaiz"() -> (w1046:dbl)
                  n580 = call <vilib>:"WPI_RobotDriveRefNum Registry Get.vi"("refnum name"="chasis") -> ("error out"=w1042:errorcluster, "RobotDriveDevRef"=w1043:T13)  [unwired: 9 in]
                  n581 = Greater Or Equal?(x=w1046, y=25.0) -> (x >= y?=w1044:bool)
                  n582 = call <vilib>:"WPI_RobotDriveTankDrive.vi"("error in (no error)"=w1042, "Right axis value"=w1041, "Left axis value"=w1041, "RobotDriveDevRef"=w1043) -> ()  [unwired: 5 in, 3 out]
                }
              }
              frame #2 {
                w1049 = 0.0 ("Motor Output")
                n583 = call <vilib>:"WPI_RobotDriveRefNum Registry Get.vi"("refnum name"="chasis") -> ("error out"=w1050:errorcluster, "RobotDriveDevRef"=w1051:T13)  [unwired: 9 in]
                n584 = call <vilib>:"WPI_RobotDriveTankDrive.vi"("error in (no error)"=w1050, "Right axis value"=w1049, "Left axis value"=w1049, "RobotDriveDevRef"=w1051) -> ()  [unwired: 5 in, 3 out]
              }
              frame #3 {
              }
            }
          }
          frame 2 {
            n585 = flat-sequence {
              tunnel: [3.0] -> w1054
              tunnel: [TRUE] -> w1053
              frame #0 {
                n586 = while {
                  stop <- w1058 stop-if-true
                  w1055 = -0.3 ("Motor Output")
                  n587 = global read "Robot Global Data.vi" "ruedaiz"() -> (w1060:dbl)
                  n588 = call <vilib>:"WPI_RobotDriveRefNum Registry Get.vi"("refnum name"="chasis") -> ("error out"=w1056:errorcluster, "RobotDriveDevRef"=w1057:T13)  [unwired: 9 in]
                  n589 = Greater Or Equal?(x=w1060, y=40.0) -> (x >= y?=w1058:bool)
                  n590 = call <vilib>:"WPI_RobotDriveTankDrive.vi"("error in (no error)"=w1056, "Right axis value"=w1055, "Left axis value"=w1055, "RobotDriveDevRef"=w1057) -> ()  [unwired: 5 in, 3 out]
                }
              }
              frame #1 {
                n591 = while {
                  stop <- FALSE stop-if-true
                  n592 = global read "Robot Global Data.vi" "stop_arduino"() -> (w1071:bool)
                  n593 = global read "Robot Global Data.vi" "full_reverse_arduino"() -> (w1068:bool)
                  n594 = global read "Robot Global Data.vi" "full_forward_arduino"() -> (w1070:bool)
                  n595 = Build Array(w1071, w1070, w1068) -> (w1069:bool[])
                  n596 = Boolean Array To Number(Boolean array=w1069) -> (number=w1067:u32)
                  n597 = case shown="1" w1067 {
                    tunnel: [0.0 0.0 -0.25 0.25] -> w1063
                    frame 0, Default {
                    }
                    frame 1 {
                    }
                    frame 2 {
                    }
                    frame 4 {
                    }
                  }
                  n598 = call <vilib>:"WPI_RobotDriveRefNum Registry Get.vi"("refnum name"="chasis") -> ("error out"=w1064:errorcluster, "RobotDriveDevRef"=w1065:T13)  [unwired: 9 in]
                  n599 = call <vilib>:"WPI_RobotDriveTankDrive.vi"("error in (no error)"=w1064, "Right axis value"=w1063, "Left axis value"=w1063, "RobotDriveDevRef"=w1065) -> ()  [unwired: 5 in, 3 out]
                }
              }
              frame #2 {
              }
            }
          }
        }
      }
    }
    frame "supreme-t" {
      n600 = while {
        shift-right: [w1080] -> _
        shift-left: 0.0 -> [w1081]
        stop <- w1079 stop-if-true
        n601 = case shown="2" w1081 {
          tunnel: [1.0 w1083 w1104] -> w1080
          tunnel: [_ _ w1103] -> w1079
          frame 0, Default {
          }
          frame 1 {
            n602 = flat-sequence {
              tunnel: [2.0] -> w1083
              frame #0 {
                w1087 = -0.2 ("Motor Output")
                n603 = call <vilib>:"WPI_RobotDriveRefNum Registry Get.vi"("refnum name"="chasis") -> ("error out"=w1088:errorcluster, "RobotDriveDevRef"=w1089:T13)  [unwired: 9 in]
                n604 = call <vilib>:"WPI_RobotDriveTankDrive.vi"("error in (no error)"=w1088, "Right axis value"=w1087, "Left axis value"=w1087, "RobotDriveDevRef"=w1089) -> ("error out"=w1086:errorcluster, "RobotDriveDevRef"=w1085:T13)  [unwired: 5 in, 1 out]
                n605 = call <vilib>:"WPI_RobotDriveDelayAndUpdateSafety.vi"("error in (no error)"=w1086, "Delay (s)"=4.0, "RobotDriveDevRef"=w1085) -> ()  [unwired: 7 in, 2 out]
              }
              frame #1 {
                w1094 = 0.8 ("Motor Output")
                n606 = call <vilib>:"WPI_RobotDriveRefNum Registry Get.vi"("refnum name"="chasis") -> ("error out"=w1095:errorcluster, "RobotDriveDevRef"=w1096:T13)  [unwired: 9 in]
                n607 = call <vilib>:"WPI_RobotDriveTankDrive.vi"("error in (no error)"=w1095, "Right axis value"=w1094, "Left axis value"=w1094, "RobotDriveDevRef"=w1096) -> ("error out"=w1092:errorcluster, "RobotDriveDevRef"=w1093:T13)  [unwired: 5 in, 1 out]
                n608 = call <vilib>:"WPI_RobotDriveDelayAndUpdateSafety.vi"("error in (no error)"=w1092, "Delay (s)"=4.0, "RobotDriveDevRef"=w1093) -> ()  [unwired: 7 in, 2 out]
              }
              frame #2 {
                w1099 = 0.0 ("Motor Output")
                n609 = call <vilib>:"WPI_RobotDriveRefNum Registry Get.vi"("refnum name"="chasis") -> ("error out"=w1100:errorcluster, "RobotDriveDevRef"=w1101:T13)  [unwired: 9 in]
                n610 = call <vilib>:"WPI_RobotDriveTankDrive.vi"("error in (no error)"=w1100, "Right axis value"=w1099, "Left axis value"=w1099, "RobotDriveDevRef"=w1101) -> ()  [unwired: 5 in, 3 out]
              }
              frame #3 {
              }
            }
          }
          frame 2 {
            n611 = flat-sequence {
              tunnel: [3.0] -> w1104
              tunnel: [TRUE] -> w1103
              frame #0 {
                w1109 = -0.3 ("Motor Output")
                n612 = call <vilib>:"WPI_RobotDriveRefNum Registry Get.vi"("refnum name"="chasis") -> ("error out"=w1110:errorcluster, "RobotDriveDevRef"=w1111:T13)  [unwired: 9 in]
                n613 = call <vilib>:"WPI_RobotDriveTankDrive.vi"("error in (no error)"=w1110, "Right axis value"=w1109, "Left axis value"=w1109, "RobotDriveDevRef"=w1111) -> ("error out"=w1107:errorcluster, "RobotDriveDevRef"=w1106:T13)  [unwired: 5 in, 1 out]
                n614 = call <vilib>:"WPI_RobotDriveDelayAndUpdateSafety.vi"("error in (no error)"=w1107, "Delay (s)"=5.0, "RobotDriveDevRef"=w1106) -> ()  [unwired: 7 in, 2 out]
              }
              frame #1 {
                n615 = while {
                  stop <- FALSE stop-if-true
                  n616 = global read "Robot Global Data.vi" "stop_arduino"() -> (w1121:bool)
                  n617 = global read "Robot Global Data.vi" "full_reverse_arduino"() -> (w1118:bool)
                  n618 = global read "Robot Global Data.vi" "full_forward_arduino"() -> (w1120:bool)
                  n619 = Build Array(w1121, w1120, w1118) -> (w1119:bool[])
                  n620 = Boolean Array To Number(Boolean array=w1119) -> (number=w1117:u32)
                  n621 = case shown="1" w1117 {
                    tunnel: [0.0 0.0 -0.25 0.25] -> w1113
                    frame 0, Default {
                    }
                    frame 1 {
                    }
                    frame 2 {
                    }
                    frame 4 {
                    }
                  }
                  n622 = call <vilib>:"WPI_RobotDriveRefNum Registry Get.vi"("refnum name"="chasis") -> ("error out"=w1114:errorcluster, "RobotDriveDevRef"=w1115:T13)  [unwired: 9 in]
                  n623 = call <vilib>:"WPI_RobotDriveTankDrive.vi"("error in (no error)"=w1114, "Right axis value"=w1113, "Left axis value"=w1113, "RobotDriveDevRef"=w1115) -> ()  [unwired: 5 in, 3 out]
                }
              }
              frame #2 {
              }
            }
          }
        }
      }
    }
  }
